vi "GVSGet Window Title Message.vi"(10 "No":i32, 11 "Kind":string) -> (0 "Control Label Off":string[](array[string]), 1 "Control Label On":string[](array[string]), 2 "Unicode String":string, 3 "Multibyte String":string, 4 "Control Name":string[](array[string]), 6 "Tip Strip":string[](array[string]))   [LabVIEW 2013]
panel:
  # "Get Window Title Message."
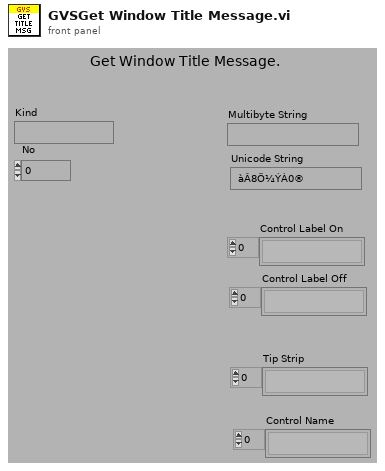
[diagram p1: front panel]
types:
  T1 = enum32{"English", "Chinese", "Korean", "Japanese", "Russian", "Chinese traditional"}
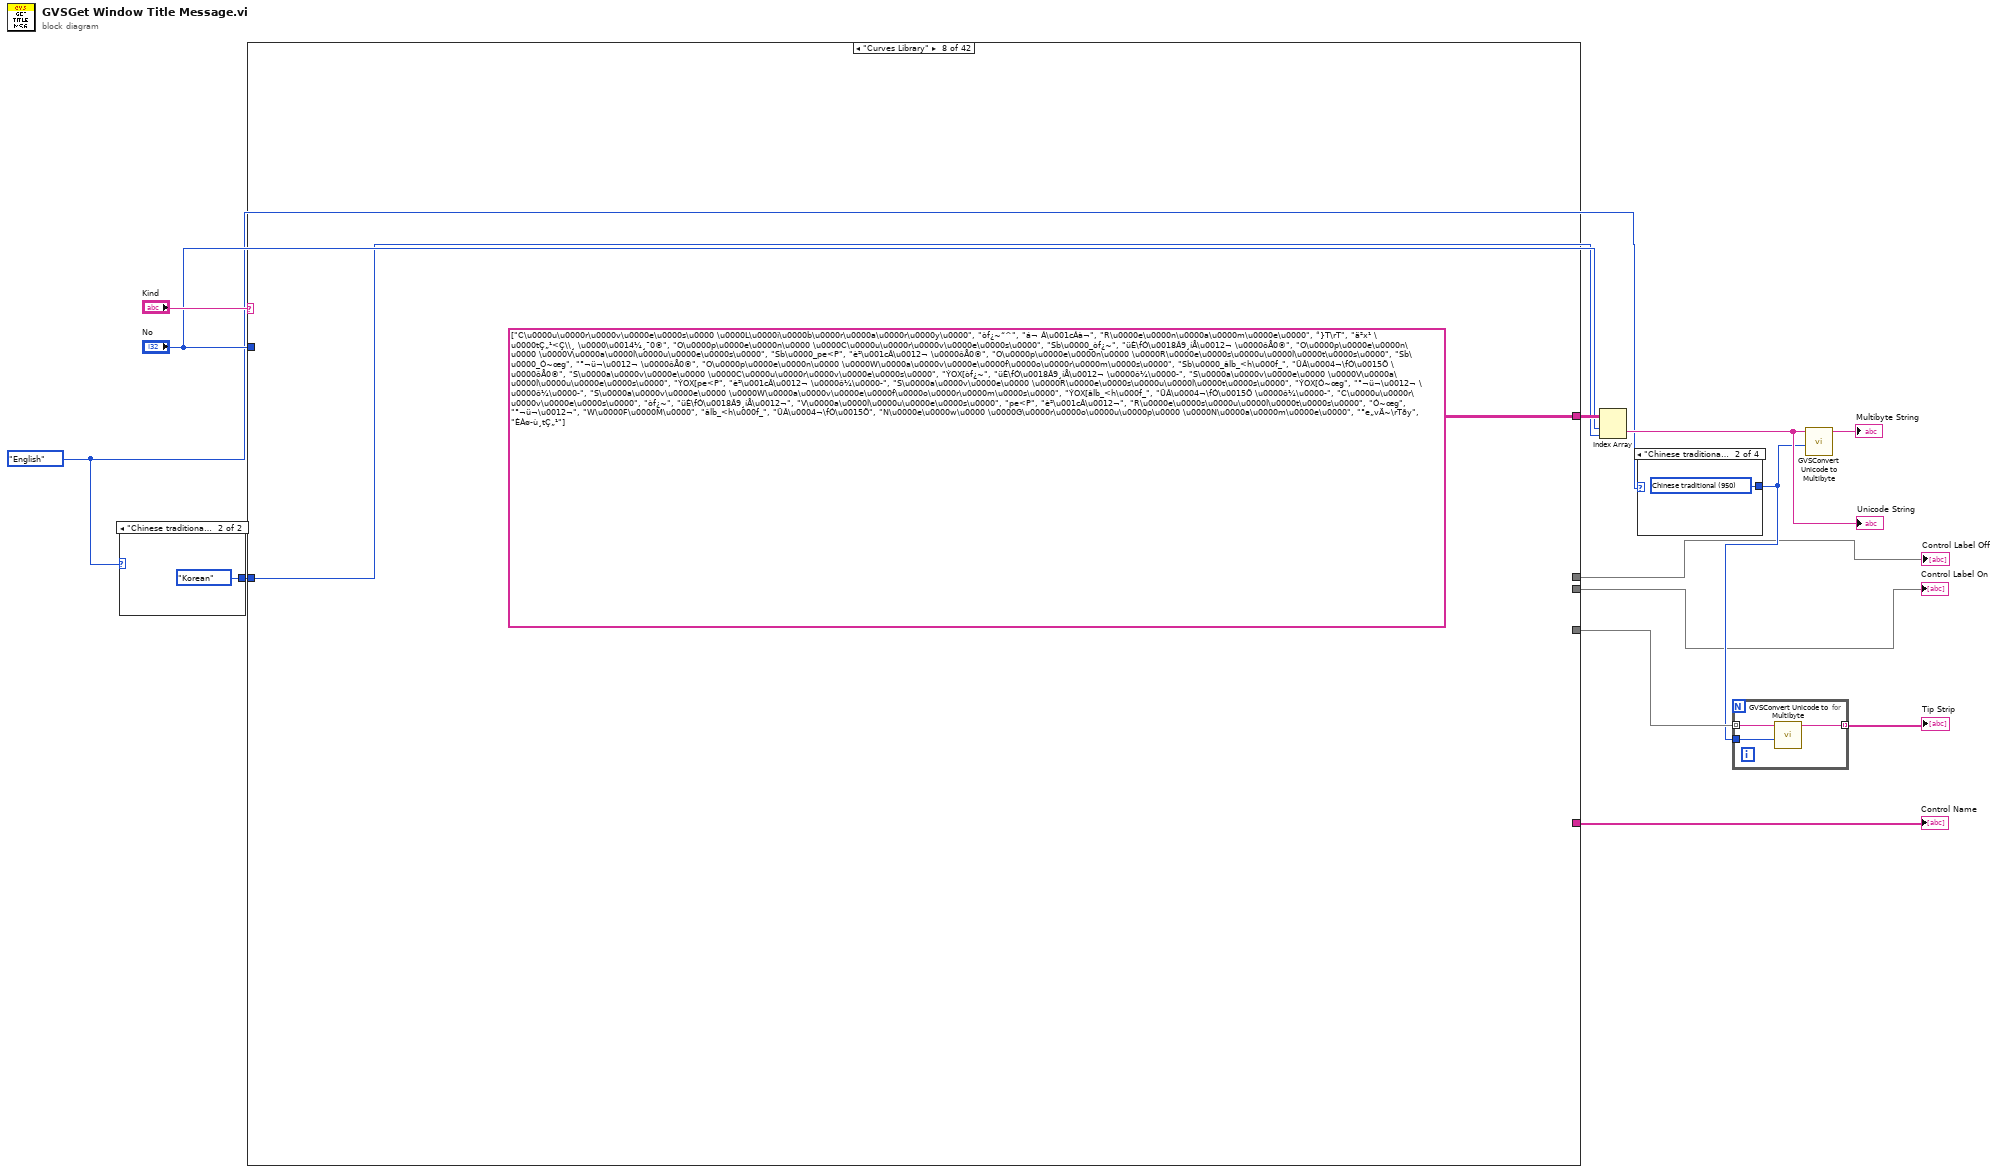
[diagram p0: block diagram]
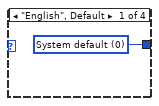
[diagram p3: hidden frame]
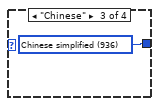
[diagram p4: hidden frame]
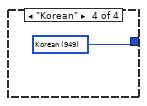
[diagram p5: hidden frame]
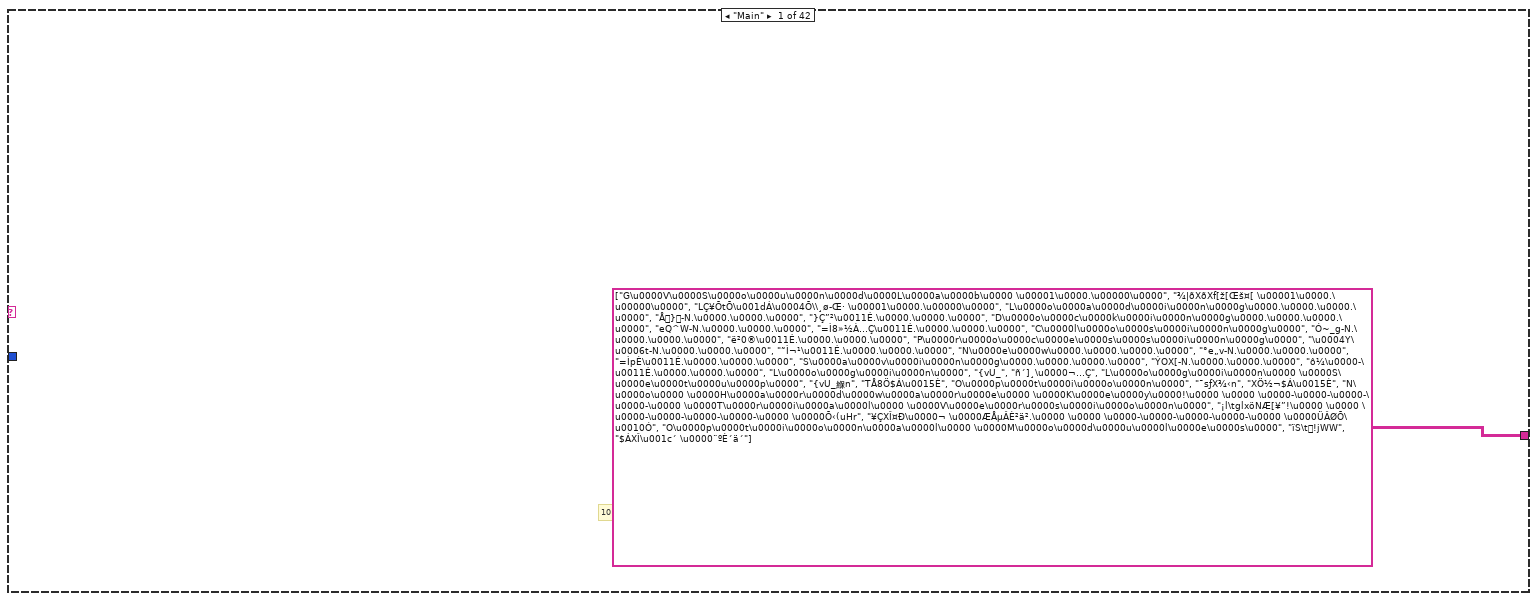
[diagram p6: hidden frame]
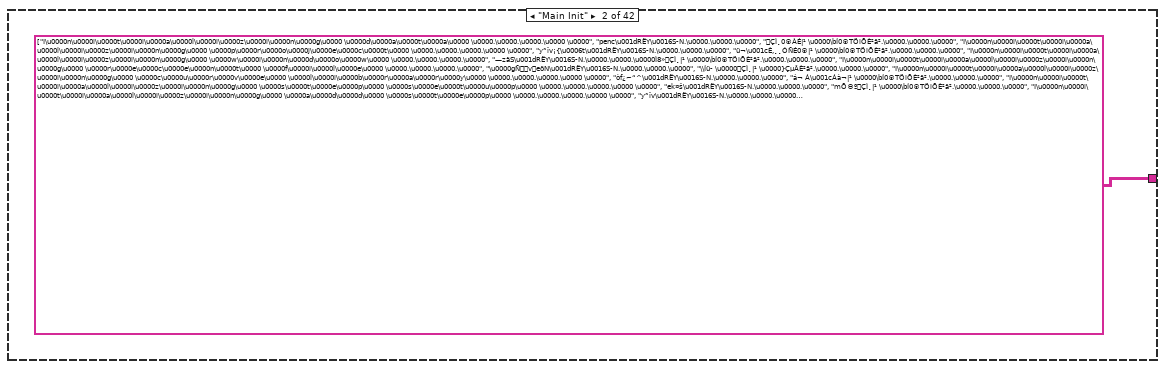
[diagram p7: hidden frame]
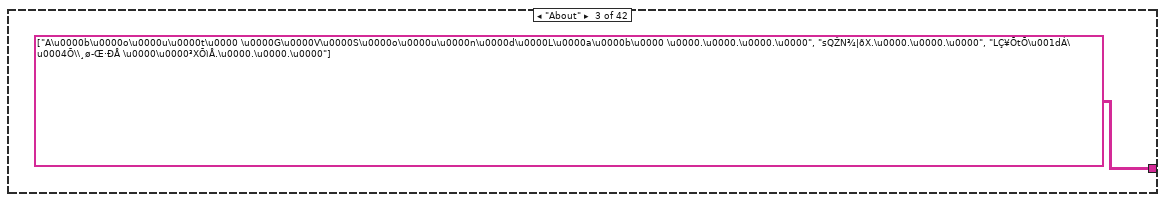
[diagram p8: hidden frame]
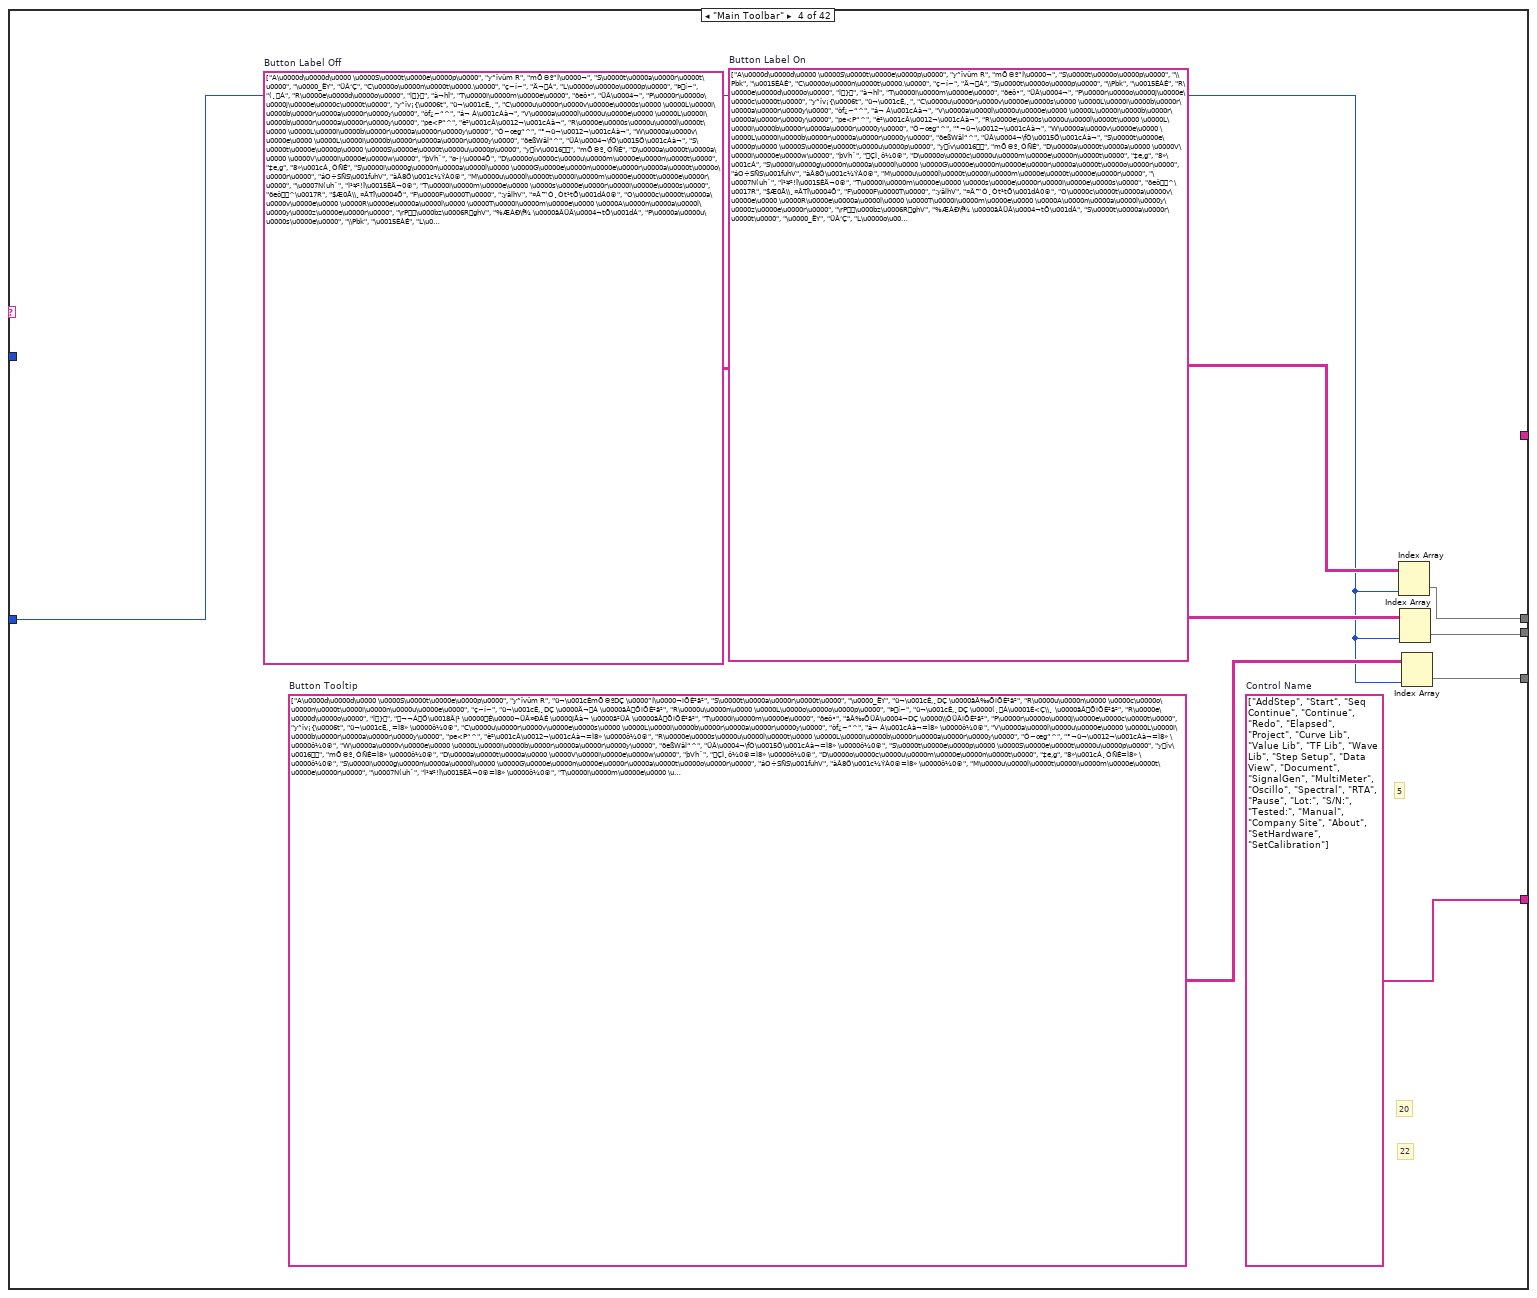
[diagram p9: hidden frame]
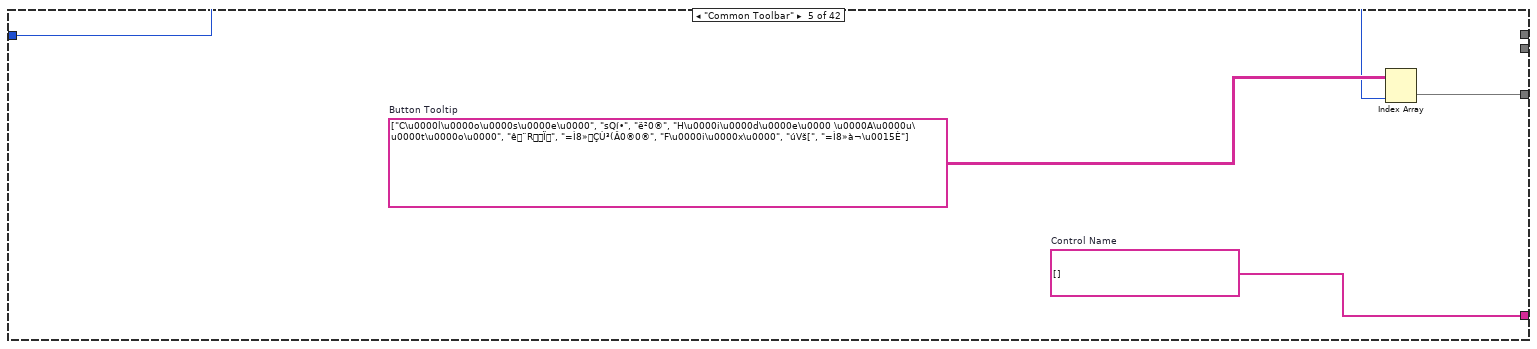
[diagram p10: hidden frame]
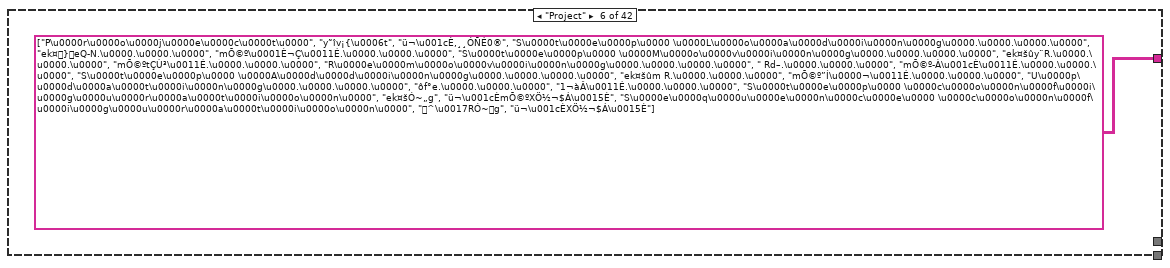
[diagram p11: hidden frame]
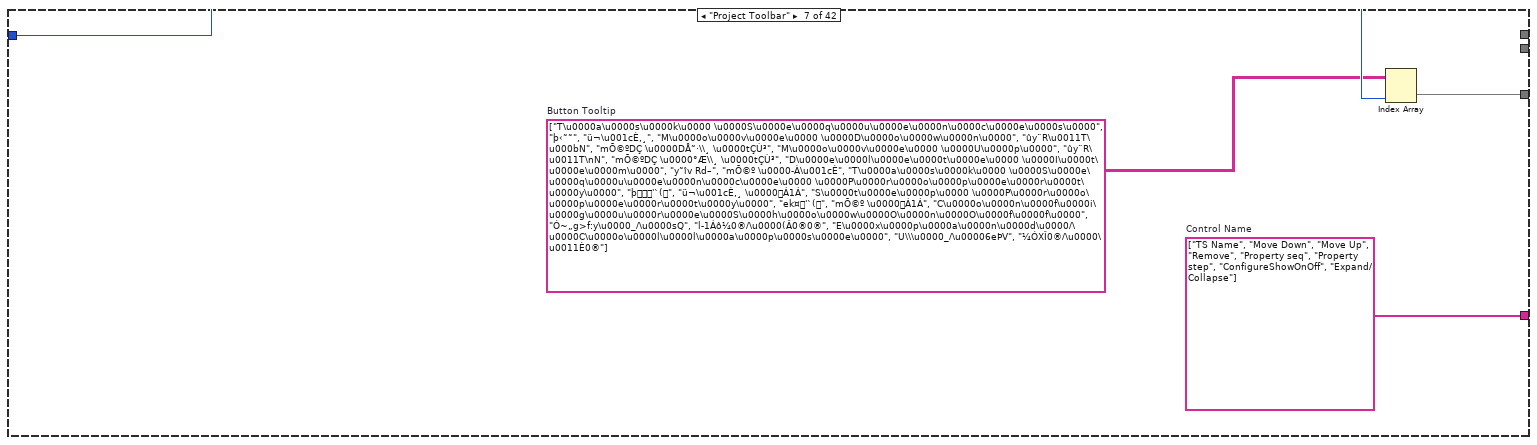
[diagram p12: hidden frame]
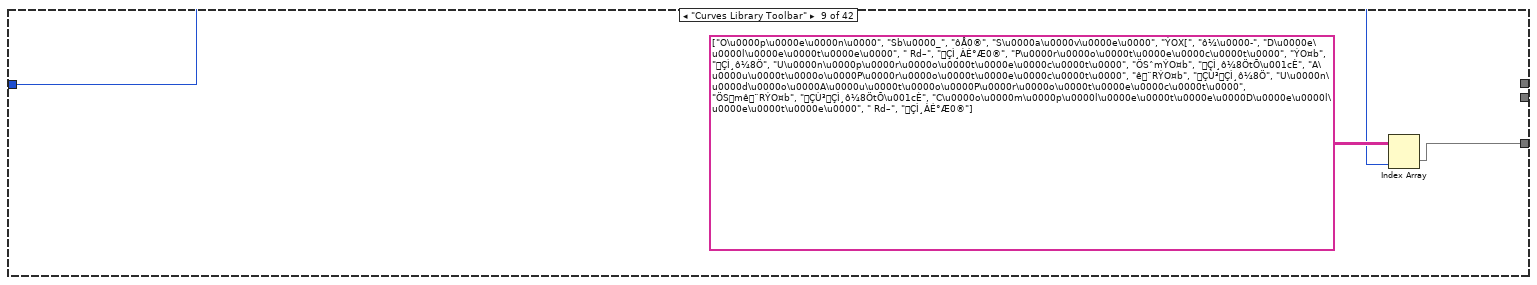
[diagram p13: hidden frame]
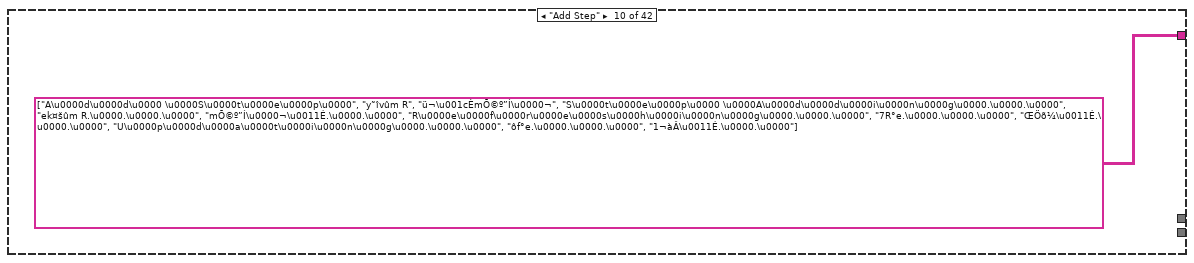
[diagram p14: hidden frame]
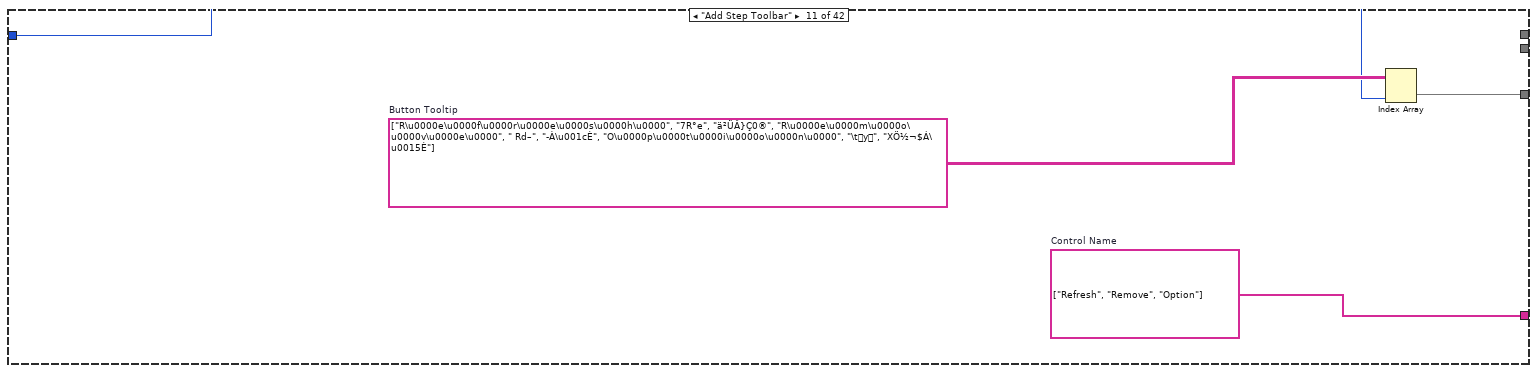
[diagram p15: hidden frame]
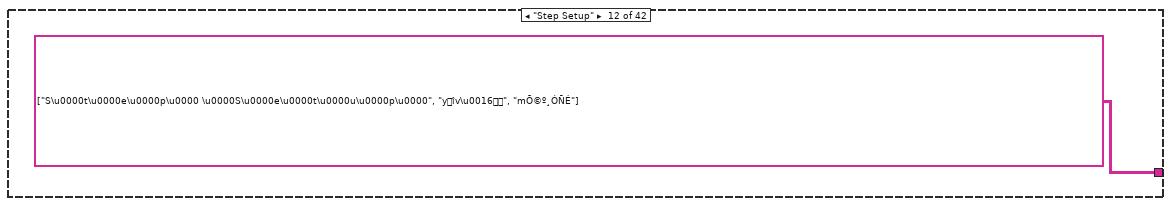
[diagram p16: hidden frame]
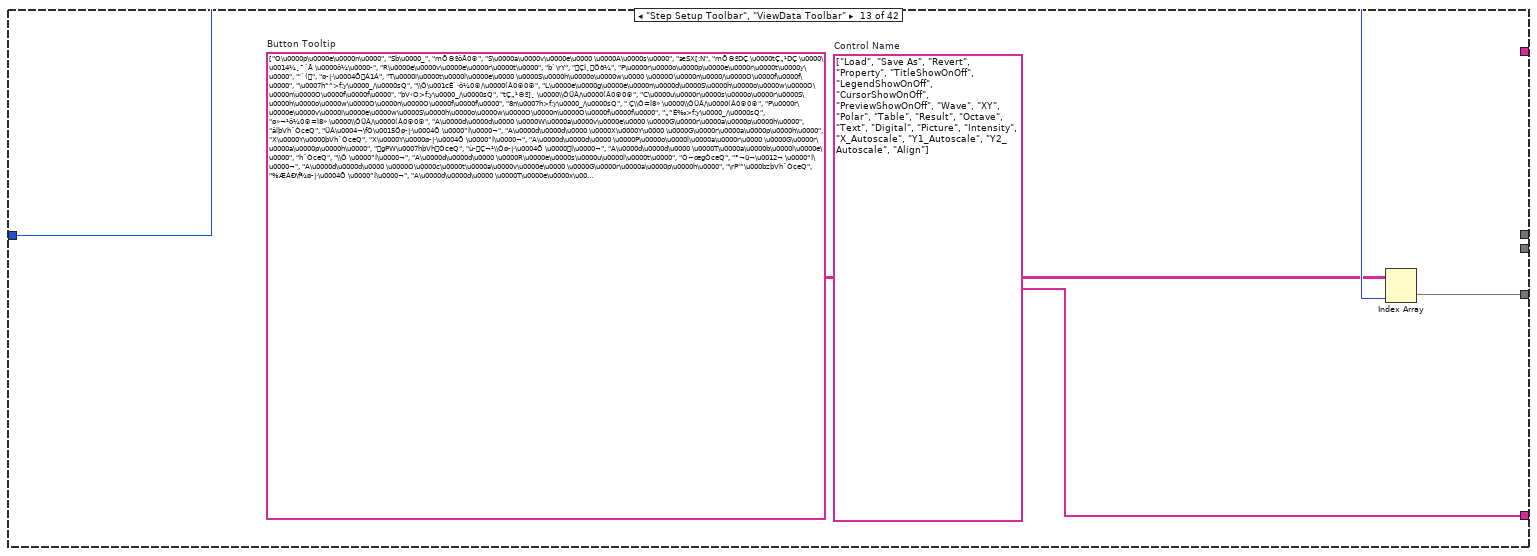
[diagram p17: hidden frame]
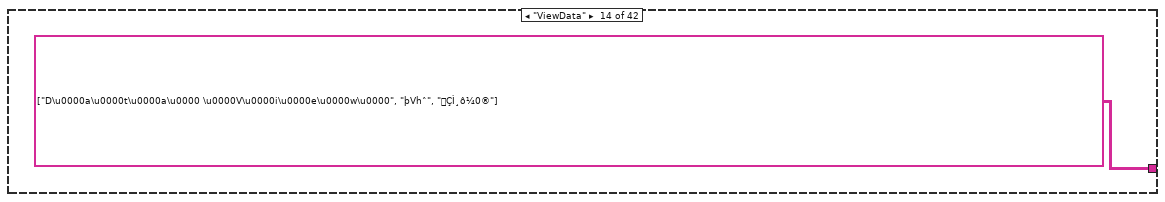
[diagram p18: hidden frame]
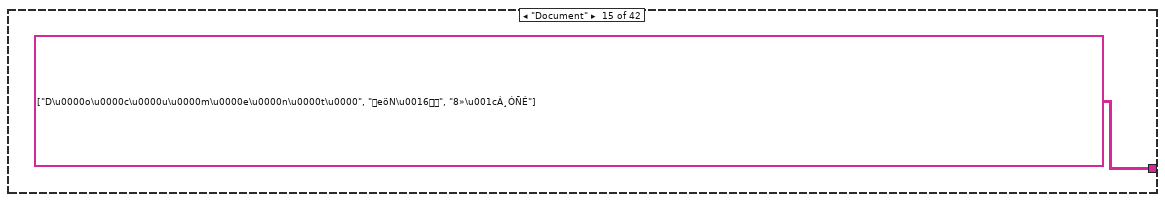
[diagram p19: hidden frame]
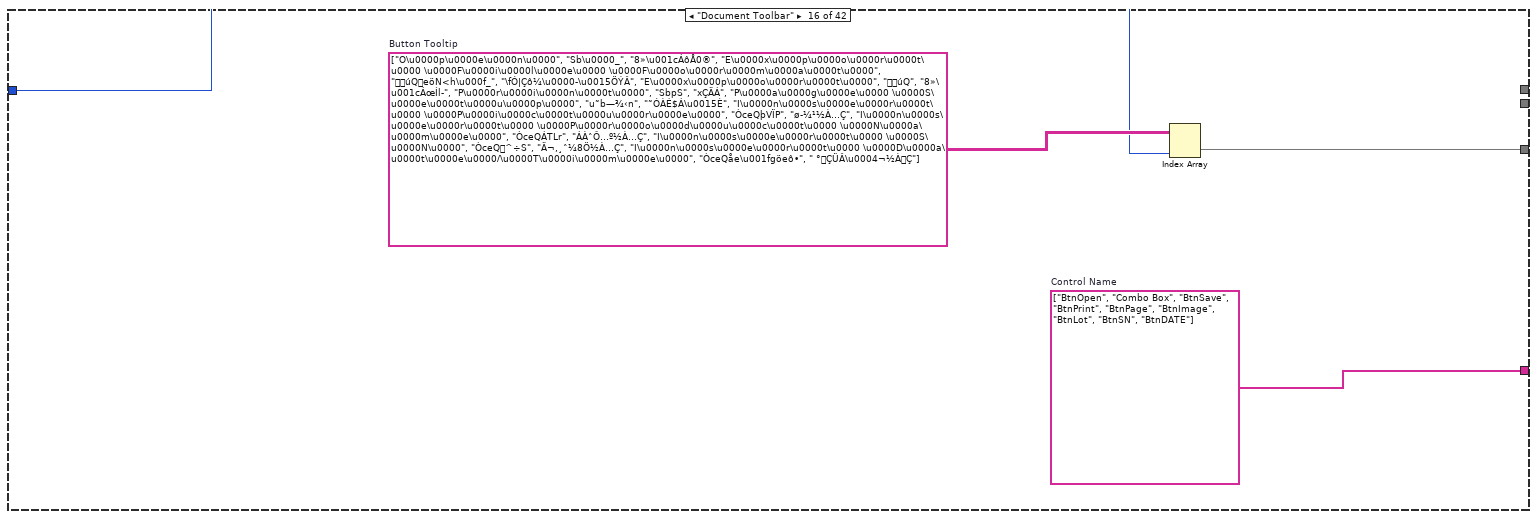
[diagram p20: hidden frame]
diagram:
  w1 = T1."English" ("Language")
  n1 = case shown="\"Chinese traditional\"" w1 {
    selector: w1 -> [w14 _]
    tunnel: [w14 T1."Korean" ("Language")] -> w2
    frame "English", Default {
    }
    frame "Chinese traditional" {
    }
  }
  n2 = case shown="\"Curves Library\"" "Kind" {
    tunnel: [string[][] [["G\u0000V\u0000S\u0000o\u0000u\u0000n\u0000d\u0000L\u0000a\u0000b\u0000 \u00001\u0000.\u00000\u0000", "¾|ðXðXf[ž[Œš¤[ \u00001\u0000.\u00000\u0000", "LÇ¥ÕtÕ\u001dÁ\u0004Õ\\¸ø­Œ· \u00001\u0000.\u00000\u0000"], ["L\u0000o\u0000a\u0000d\u0000i\u0000n\u0000g\u0000.\u0000.\u0000.\u0000", "Å}-N.\u0000.\u0000.\u0000", "}Ç”²\u0011É.\u0000.\u0000.\u0000"], ["D\u0000o\u0000c\u0000k\u0000i\u0000n\u0000g\u0000.\u0000.\u0000.\u0000", "eQ^W-N.\u0000.\u0000.\u0000", "=Ì8»½À…Ç\u0011É.\u0000.\u0000.\u0000"], ["C\u0000l\u0000o\u0000s\u0000i\u0000n\u0000g\u0000", "Ó~_g-N.\u0000.\u0000.\u0000", "ë²0®\u0011É.\u0000.\u0000.\u0000"], ["P\u0000r\u0000o\u0000c\u0000e\u0000s\u0000s\u0000i\u0000n\u0000g\u0000", "\u0004Y\u0006t-N.\u0000.\u0000.\u0000", "˜Ì¬¹\u0011É.\u0000.\u0000.\u0000"], ["N\u0000e\u0000w\u0000.\u0000.\u0000.\u0000", "°e„v-N.\u0000.\u0000.\u0000", "=ÌpÈ\u0011É.\u0000.\u0000.\u0000"], ["S\u0000a\u0000v\u0000i\u0000n\u0000g\u0000.\u0000.\u0000.\u0000", "ÝOX[-N.\u0000.\u0000.\u0000", "ô¼\u0000­\u0011É.\u0000.\u0000.\u0000"], ["L\u0000o\u0000g\u0000i\u0000n\u0000", "{vU_", "ñ´]¸\u0000¬…Ç"], ["L\u0000o\u0000g\u0000i\u0000n\u0000 \u0000S\u0000e\u0000t\u0000u\u0000p\u0000", "{vU_緥n", "TÅ8Ö$Á\u0015È"], ["O\u0000p\u0000t\u0000i\u0000o\u0000n\u0000", "¯sƒX¾‹n", "XÖ½¬$Á\u0015È"], ["N\u0000o\u0000 \u0000H\u0000a\u0000r\u0000d\u0000w\u0000a\u0000r\u0000e\u0000 \u0000K\u0000e\u0000y\u0000!\u0000 \u0000 \u0000-\u0000-\u0000-\u0000-\u0000 \u0000T\u0000r\u0000i\u0000a\u0000l\u0000 \u0000V\u0000e\u0000r\u0000s\u0000i\u0000o\u0000n\u0000", "¡l\tglxöNÆ[¥”!\u0000 \u0000 \u0000-\u0000-\u0000-\u0000-\u0000 \u0000Õ‹(uHr", "¥ÇXÎ¤Ð\u0000¬ \u0000ÆÅµÂÈ²ä².\u0000 \u0000 \u0000-\u0000-\u0000-\u0000-\u0000 \u0000ÜÂØÕ\u0010Ó"], ["O\u0000p\u0000t\u0000i\u0000o\u0000n\u0000a\u0000l\u0000 \u0000M\u0000o\u0000d\u0000u\u0000l\u0000e\u0000s\u0000", "ïS\t!jWW", "$ÁXÎ\u001c´ \u0000¨ºÈ´ä´"]] string[][] [["I\u0000n\u0000i\u0000t\u0000i\u0000a\u0000l\u0000i\u0000z\u0000i\u0000n\u0000g\u0000 \u0000d\u0000a\u0000t\u0000a\u0000 \u0000.\u0000.\u0000.\u0000 \u0000", "penc\u001dRËY\u0016S-N.\u0000.\u0000.\u0000", "ÇÌ¸0®ÀÉ|¹ \u0000\bÍ0®TÖiÕÈ²ä².\u0000.\u0000.\u0000"], ["I\u0000n\u0000i\u0000t\u0000i\u0000a\u0000l\u0000i\u0000z\u0000i\u0000n\u0000g\u0000 \u0000p\u0000r\u0000o\u0000j\u0000e\u0000c\u0000t\u0000 \u0000.\u0000.\u0000.\u0000 \u0000", "y˜îv¡{\u0006t\u001dRËY\u0016S-N.\u0000.\u0000.\u0000", "ü¬\u001cÈ,¸¸ÓÑÉ0®|¹ \u0000\bÍ0®TÖiÕÈ²ä².\u0000.\u0000.\u0000"], ["I\u0000n\u0000i\u0000t\u0000i\u0000a\u0000l\u0000i\u0000z\u0000i\u0000n\u0000g\u0000 \u0000w\u0000i\u0000n\u0000d\u0000o\u0000w\u0000 \u0000.\u0000.\u0000.\u0000", "—zãS\u001dRËY\u0016S-N.\u0000.\u0000.\u0000", "=Ì8»ÇÌ¸|¹ \u0000\bÍ0®TÖiÕÈ²ä².\u0000.\u0000.\u0000"], ["I\u0000n\u0000i\u0000t\u0000i\u0000a\u0000l\u0000i\u0000z\u0000i\u0000n\u0000g\u0000 \u0000r\u0000e\u0000c\u0000e\u0000n\u0000t\u0000 \u0000f\u0000i\u0000l\u0000e\u0000 \u0000.\u0000.\u0000.\u0000", "\u0000gÑveöN\u001dRËY\u0016S-N.\u0000.\u0000.\u0000", "\\Íü­ \u0000ÇÌ¸|¹ \u0000}ÇµÂÈ²ä².\u0000.\u0000.\u0000"], ["I\u0000n\u0000i\u0000t\u0000i\u0000a\u0000l\u0000i\u0000z\u0000i\u0000n\u0000g\u0000 \u0000c\u0000u\u0000r\u0000v\u0000e\u0000 \u0000l\u0000i\u0000b\u0000r\u0000a\u0000r\u0000y\u0000 \u0000.\u0000.\u0000.\u0000 \u0000", "òf¿~“^\u001dRËY\u0016S-N.\u0000.\u0000.\u0000", "á¬ Á\u001cÁà¬|¹ \u0000\bÍ0®TÖiÕÈ²ä².\u0000.\u0000.\u0000"], ["I\u0000n\u0000i\u0000t\u0000i\u0000a\u0000l\u0000i\u0000z\u0000i\u0000n\u0000g\u0000 \u0000s\u0000t\u0000e\u0000p\u0000 \u0000s\u0000e\u0000t\u0000u\u0000p\u0000 \u0000.\u0000.\u0000.\u0000 \u0000", "ek¤š\u001dRËY\u0016S-N.\u0000.\u0000.\u0000", "mÕ©ºÇÌ¸|¹ \u0000\bÍ0®TÖiÕÈ²ä².\u0000.\u0000.\u0000"], ["I\u0000n\u0000i\u0000t\u0000i\u0000a\u0000l\u0000i\u0000z\u0000i\u0000n\u0000g\u0000 \u0000a\u0000d\u0000d\u0000 \u0000s\u0000t\u0000e\u0000p\u0000 \u0000.\u0000.\u0000.\u0000 \u0000", "y˜îv\u001dRËY\u0016S-N.\u0000.\u0000.\u0000", "mÕ©ºÍ\u0000¬ÇÌ¸|¹ \u0000\u0001È¬ÇiÕÈ²ä².\u0000.\u0000.\u0000"], ["I\u0000n\u0000i\u0000t\u0000i\u0000a\u0000l\u0000i\u0000z\u0000i\u0000n\u0000g\u0000 \u0000t\u0000a\u0000s\u0000k\u0000 \u0000s\u0000e\u0000q\u0000u\u0000e\u0000n\u0000c\u0000e\u0000 \u0000.\u0000.\u0000.\u0000", "^\u0017R\u001dRËY\u0016S-N.\u0000.\u0000.\u0000", "ü¬\u001cÈ,¸DÇ \u0000\bÍ0®TÖiÕÈ²ä².\u0000.\u0000.\u0000"], ["I\u0000n\u0000i\u0000t\u0000i\u0000a\u0000l\u0000i\u0000z\u0000i\u0000n\u0000g\u0000 \u0000v\u0000i\u0000r\u0000t\u0000u\u0000a\u0000l\u0000 \u0000d\u0000a\u0000t\u0000a\u0000 \u0000.\u0000.\u0000.\u0000", "—zãS\u001dRËY\u0016S-N.\u0000.\u0000.\u0000", "\u0000¬ÁÀ=Ì8»ÇÌ¸|¹ \u0000\u0001È¬ÇiÕÈ²ä².\u0000.\u0000.\u0000"], ["I\u0000n\u0000i\u0000t\u0000i\u0000a\u0000l\u0000i\u0000z\u0000i\u0000n\u0000g\u0000 \u0000O\u0000p\u0000e\u0000r\u0000a\u0000t\u0000o\u0000r\u0000 \u0000.\u0000.\u0000.\u0000 \u0000", "Íd\\O\u001dRËY\u0016S-N.\u0000.\u0000.\u0000", "äÂÜÂ\u0004¬Ä³l­|¹ \u0000\bÍ0®TÖiÕÈ²ä².\u0000.\u0000.\u0000"], ["L\u0000o\u0000a\u0000d\u0000i\u0000n\u0000g\u0000 \u0000m\u0000a\u0000i\u0000n\u0000 \u0000w\u0000i\u0000n\u0000d\u0000o\u0000w\u0000 \u0000.\u0000.\u0000.\u0000", ";N—zãS\u001dRËY\u0016S-N.\u0000.\u0000.\u0000", "üÈ\u0004Õ\\¸ø­Œ·DÇ \u0000\u0001È¬ÇXÕà¬ˆÇµÂÈ²ä².\u0000.\u0000.\u0000"], ["L\u0000o\u0000a\u0000d\u0000i\u0000n\u0000g\u0000 \u0000m\u0000a\u0000i\u0000n\u0000 \u0000w\u0000i\u0000n\u0000d\u0000o\u0000w\u0000 \u0000.\u0000 \u0000.\u0000", ";N—zãS\u001dRËY\u0016S-N.\u0000 \u0000.\u0000", "üÈ\u0004Õ\\¸ø­Œ·DÇ \u0000\u0001È¬ÇXÕà¬ˆÇµÂÈ²ä².\u0000 \u0000.\u0000"], ["L\u0000o\u0000a\u0000d\u0000i\u0000n\u0000g\u0000 \u0000m\u0000a\u0000i\u0000n\u0000 \u0000w\u0000i\u0000n\u0000d\u0000o\u0000w\u0000 \u0000.\u0000.\u0000 \u0000", ";N—zãS\u001dRËY\u0016S-N.\u0000.\u0000 \u0000", "üÈ\u0004Õ\\¸ø­Œ·DÇ \u0000\u0001È¬ÇXÕà¬ˆÇµÂÈ²ä².\u0000.\u0000 \u0000"]] string[][] [["A\u0000b\u0000o\u0000u\u0000t\u0000 \u0000G\u0000V\u0000S\u0000o\u0000u\u0000n\u0000d\u0000L\u0000a\u0000b\u0000 \u0000.\u0000.\u0000.\u0000", "sQŽN¾|ðX.\u0000.\u0000.\u0000", "LÇ¥ÕtÕ\u001dÁ\u0004Õ\\¸ø­Œ·ÐÅ \u0000\u0000³XÕìÅ.\u0000.\u0000.\u0000"]] _ _ string[][] [["P\u0000r\u0000o\u0000j\u0000e\u0000c\u0000t\u0000", "y˜îv¡{\u0006t", "ü¬\u001cÈ,¸¸ÓÑÉ0®"], ["S\u0000t\u0000e\u0000p\u0000 \u0000L\u0000o\u0000a\u0000d\u0000i\u0000n\u0000g\u0000.\u0000.\u0000.\u0000", "ek¤}eQ-N.\u0000.\u0000.\u0000", "mÕ©º\u0001È¬Ç\u0011É.\u0000.\u0000.\u0000"], ["S\u0000t\u0000e\u0000p\u0000 \u0000M\u0000o\u0000v\u0000i\u0000n\u0000g\u0000.\u0000.\u0000.\u0000", "ek¤šûy¨R.\u0000.\u0000.\u0000", "mÕ©ºtÇÙ³\u0011É.\u0000.\u0000.\u0000"], ["R\u0000e\u0000m\u0000o\u0000v\u0000i\u0000n\u0000g\u0000.\u0000.\u0000.\u0000", " Rd–.\u0000.\u0000.\u0000", "mÕ©º­À\u001cÈ\u0011É.\u0000.\u0000.\u0000"], ["S\u0000t\u0000e\u0000p\u0000 \u0000A\u0000d\u0000d\u0000i\u0000n\u0000g\u0000.\u0000.\u0000.\u0000", "ek¤šûm R.\u0000.\u0000.\u0000", "mÕ©º”Í\u0000¬\u0011É.\u0000.\u0000.\u0000"], ["U\u0000p\u0000d\u0000a\u0000t\u0000i\u0000n\u0000g\u0000.\u0000.\u0000.\u0000", "ôf°e.\u0000.\u0000.\u0000", "1¬àÂ\u0011É.\u0000.\u0000.\u0000"], ["S\u0000t\u0000e\u0000p\u0000 \u0000c\u0000o\u0000n\u0000f\u0000i\u0000g\u0000u\u0000r\u0000a\u0000t\u0000i\u0000o\u0000n\u0000", "ek¤šÓ~„g", "ü¬\u001cÈmÕ©ºXÖ½¬$Á\u0015È"], ["S\u0000e\u0000q\u0000u\u0000e\u0000n\u0000c\u0000e\u0000 \u0000c\u0000o\u0000n\u0000f\u0000i\u0000g\u0000u\u0000r\u0000a\u0000t\u0000i\u0000o\u0000n\u0000", "^\u0017RÓ~g", "ü¬\u001cÈXÖ½¬$Á\u0015È"]] _ string[][] [["C\u0000u\u0000r\u0000v\u0000e\u0000s\u0000 \u0000L\u0000i\u0000b\u0000r\u0000a\u0000r\u0000y\u0000", "òf¿~“^", "á¬ Á\u001cÁà¬"], ["R\u0000e\u0000n\u0000a\u0000m\u0000e\u0000", "͑}T\rT", "ä²x¹ \u0000tÇ„¹<Ç\\¸ \u0000\u0014¼¸¯0®"], ["O\u0000p\u0000e\u0000n\u0000 \u0000C\u0000u\u0000r\u0000v\u0000e\u0000s\u0000", "Sb\u0000_òf¿~", "üÈ\fÓ\u0018Â9¸íÅ\u0012¬ \u0000ôÅ0®"], ["O\u0000p\u0000e\u0000n\u0000 \u0000V\u0000a\u0000l\u0000u\u0000e\u0000s\u0000", "Sb\u0000_pe<P", "è²\u001cÂ\u0012¬ \u0000ôÅ0®"], ["O\u0000p\u0000e\u0000n\u0000 \u0000R\u0000e\u0000s\u0000u\u0000l\u0000t\u0000s\u0000", "Sb\u0000_Ó~œg", "°¬ü¬\u0012¬ \u0000ôÅ0®"], ["O\u0000p\u0000e\u0000n\u0000 \u0000W\u0000a\u0000v\u0000e\u0000f\u0000o\u0000r\u0000m\u0000s\u0000", "Sb\u0000_âlb_<h\u000f_", "ÜÂ\u0004¬\fÓ\u0015Ö \u0000ôÅ0®"], ["S\u0000a\u0000v\u0000e\u0000 \u0000C\u0000u\u0000r\u0000v\u0000e\u0000s\u0000", "ÝOX[òf¿~", "üÈ\fÓ\u0018Â9¸íÅ\u0012¬ \u0000ô¼\u0000­"], ["S\u0000a\u0000v\u0000e\u0000 \u0000V\u0000a\u0000l\u0000u\u0000e\u0000s\u0000", "ÝOX[pe<P", "è²\u001cÂ\u0012¬ \u0000ô¼\u0000­"], ["S\u0000a\u0000v\u0000e\u0000 \u0000R\u0000e\u0000s\u0000u\u0000l\u0000t\u0000s\u0000", "ÝOX[Ó~œg", "°¬ü¬\u0012¬ \u0000ô¼\u0000­"], ["S\u0000a\u0000v\u0000e\u0000 \u0000W\u0000a\u0000v\u0000e\u0000f\u0000o\u0000r\u0000m\u0000s\u0000", "ÝOX[âlb_<h\u000f_", "ÜÂ\u0004¬\fÓ\u0015Ö \u0000ô¼\u0000­"], ["C\u0000u\u0000r\u0000v\u0000e\u0000s\u0000", "òf¿~", "üÈ\fÓ\u0018Â9¸íÅ\u0012¬"], ["V\u0000a\u0000l\u0000u\u0000e\u0000s\u0000", "pe<P", "è²\u001cÂ\u0012¬"], ["R\u0000e\u0000s\u0000u\u0000l\u0000t\u0000s\u0000", "Ó~œg", "°¬ü¬\u0012¬"], ["W\u0000F\u0000M\u0000", "âlb_<h\u000f_", "ÜÂ\u0004¬\fÓ\u0015Ö"], ["N\u0000e\u0000w\u0000 \u0000G\u0000r\u0000o\u0000u\u0000p\u0000 \u0000N\u0000a\u0000m\u0000e\u0000", "°e„vÄ~\rTðy", "ÈÀø­ù¸tÇ„¹"]] _ string[][] [["A\u0000d\u0000d\u0000 \u0000S\u0000t\u0000e\u0000p\u0000", "y˜îvûm R", "ü¬\u001cÈmÕ©º”Í\u0000¬"], ["S\u0000t\u0000e\u0000p\u0000 \u0000A\u0000d\u0000d\u0000i\u0000n\u0000g\u0000.\u0000.\u0000", "ek¤šûm R.\u0000.\u0000.\u0000", "mÕ©º”Í\u0000¬\u0011É.\u0000.\u0000"], ["R\u0000e\u0000f\u0000r\u0000e\u0000s\u0000h\u0000i\u0000n\u0000g\u0000.\u0000.\u0000", "7R°e.\u0000.\u0000.\u0000", "ŒÖõ¼\u0011É.\u0000.\u0000"], ["U\u0000p\u0000d\u0000a\u0000t\u0000i\u0000n\u0000g\u0000.\u0000.\u0000", "ôf°e.\u0000.\u0000.\u0000", "1¬àÂ\u0011É.\u0000.\u0000"]] _ string[][] [["S\u0000t\u0000e\u0000p\u0000 \u0000S\u0000e\u0000t\u0000u\u0000p\u0000", "yîv\u0016", "mÕ©º¸ÓÑÉ"]] _ string[][] [["D\u0000a\u0000t\u0000a\u0000 \u0000V\u0000i\u0000e\u0000w\u0000", "þVhˆ", "ÇÌ¸ô¼0®"]] string[][] [["D\u0000o\u0000c\u0000u\u0000m\u0000e\u0000n\u0000t\u0000", "eöN\u0016", "8»\u001cÁ¸ÓÑÉ"]] _ string[][] [["R\u0000u\u0000n\u0000 \u0000P\u0000r\u0000o\u0000j\u0000e\u0000c\u0000t\u0000", "yîvÐL", "ü¬\u001cÈ,¸ \u0000äÂ‰Õ"]] string[][] [["W\u0000a\u0000v\u0000e\u0000 \u0000G\u0000r\u0000a\u0000p\u0000h\u0000", "âlþVhˆ", "ÜÂ\u0004¬\fÓ\u0015Öø­|·\u0004Õ"], ["W\u0000a\u0000v\u0000e\u0000 \u0000G\u0000r\u0000a\u0000p\u0000h\u0000 \u0000P\u0000r\u0000o\u0000p\u0000e\u0000r\u0000t\u0000y\u0000", "âlþVhˆ^\\'`", "ÜÂ\u0004¬\fÓ\u0015Öø­|·\u0004ÕÁ1Á"]] string[][] [["X\u0000Y\u0000 \u0000G\u0000r\u0000a\u0000p\u0000h\u0000", "X\u0000Y\u0000þVhˆ", "X\u0000Y\u0000ø­|·\u0004Õ"], ["X\u0000Y\u0000 \u0000G\u0000r\u0000a\u0000p\u0000h\u0000 \u0000P\u0000r\u0000o\u0000p\u0000e\u0000r\u0000t\u0000y\u0000", "X\u0000Y\u0000þVhˆ^\\'`", "X\u0000Y\u0000ø­|·\u0004ÕÁ1Á"]] string[][] [["D\u0000i\u0000g\u0000i\u0000t\u0000a\u0000l\u0000 \u0000G\u0000r\u0000a\u0000p\u0000h\u0000", "peW[þVhˆ", "\u0018ÂÇàÂ8Öø­|·\u0004Õ"], ["D\u0000i\u0000g\u0000i\u0000t\u0000a\u0000l\u0000 \u0000G\u0000r\u0000a\u0000p\u0000h\u0000 \u0000P\u0000r\u0000o\u0000p\u0000e\u0000r\u0000t\u0000y\u0000", "peW[þVhˆ^\\'`", "\u0018ÂÇàÂ8Öø­|·\u0004ÕÁ1Á"]] string[][] [["O\u0000c\u0000t\u0000a\u0000v\u0000e\u0000 \u0000G\u0000r\u0000a\u0000p\u0000h\u0000", "\rP‘˜\u000bzþVhˆ", "%ÆÀÐ\f¾ø­|·\u0004Õ"], ["O\u0000c\u0000t\u0000a\u0000v\u0000e\u0000 \u0000G\u0000r\u0000a\u0000p\u0000h\u0000 \u0000P\u0000r\u0000o\u0000p\u0000e\u0000r\u0000t\u0000y\u0000", "\rP‘˜\u000bzþVhˆ^\\'`", "%ÆÀÐ\f¾ø­|·\u0004ÕÁ1Á"]] string[][] [["P\u0000o\u0000l\u0000a\u0000r\u0000 \u0000G\u0000r\u0000a\u0000p\u0000h\u0000", "gPW\u0007hþVh", "ù­Ç¬¹\\Ôø­|·\u0004Õ"], ["P\u0000o\u0000l\u0000a\u0000r\u0000 \u0000G\u0000r\u0000a\u0000p\u0000h\u0000 \u0000P\u0000r\u0000o\u0000p\u0000e\u0000r\u0000t\u0000y\u0000 \u0000", "gPW\u0007hþVh^\\'`", "ù­Ç¬¹\\Ôø­|·\u0004ÕÁ1Á"]] string[][] [["T\u0000e\u0000x\u0000t\u0000", ",g‡e", "ø¼8»"], ["T\u0000e\u0000x\u0000t\u0000 \u0000P\u0000r\u0000o\u0000p\u0000e\u0000r\u0000t\u0000y\u0000", ",g‡e^\\'`", "ø¼8»Á1Á"]] string[][] [["T\u0000a\u0000b\u0000l\u0000e\u0000 \u0000G\u0000r\u0000a\u0000p\u0000h\u0000", "hˆ", "\\Ô"], ["T\u0000a\u0000b\u0000l\u0000e\u0000 \u0000G\u0000r\u0000a\u0000p\u0000h\u0000 \u0000P\u0000r\u0000o\u0000p\u0000e\u0000r\u0000t\u0000y\u0000", "hˆ^\\'`", "\\ÔÁ1Á"]] string[][] [["P\u0000i\u0000c\u0000t\u0000u\u0000r\u0000e\u0000 \u0000G\u0000r\u0000a\u0000p\u0000h\u0000", "þVÏP", "ø­¼¹"], ["P\u0000i\u0000c\u0000t\u0000u\u0000r\u0000e\u0000 \u0000G\u0000r\u0000a\u0000p\u0000h\u0000 \u0000P\u0000r\u0000o\u0000p\u0000e\u0000r\u0000t\u0000y\u0000", "þVÏP^\\'`", "ø­¼¹Á1Á"]] string[][] [["R\u0000e\u0000s\u0000u\u0000l\u0000t\u0000 \u0000G\u0000r\u0000a\u0000p\u0000h\u0000", "Ó~œg", "°¬ü¬\u0012¬"], ["R\u0000e\u0000s\u0000u\u0000l\u0000t\u0000 \u0000G\u0000r\u0000a\u0000p\u0000h\u0000 \u0000P\u0000r\u0000o\u0000p\u0000e\u0000r\u0000t\u0000y\u0000", "Ó~œg^\\'`", "°¬ü¬\u0012¬Á1Á"]] string[][] [["I\u0000n\u0000t\u0000e\u0000n\u0000s\u0000i\u0000t\u0000y\u0000 \u0000G\u0000r\u0000a\u0000p\u0000h\u0000", "Æ[¦^þVhˆ", "\u0000¼Ä³ø­|·\u0004Õ"], ["I\u0000n\u0000t\u0000e\u0000n\u0000s\u0000i\u0000t\u0000y\u0000 \u0000G\u0000r\u0000a\u0000p\u0000h\u0000 \u0000P\u0000r\u0000o\u0000p\u0000e\u0000r\u0000t\u0000y\u0000", "Æ[¦^þVhˆ^\\'`", "\u0000¼Ä³ø­|·\u0004ÕÁ1Á"]] string[][] [["C\u0000h\u0000a\u0000n\u0000n\u0000e\u0000l\u0000 \u0000E\u0000d\u0000i\u0000t\u0000o\u0000r\u0000", "\u001aS\u0016", "µÑ\\¸¸ÓÑÉ"]] string[][] [["C\u0000a\u0000l\u0000i\u0000b\u0000r\u0000a\u0000t\u0000i\u0000o\u0000n\u0000 \u0000P\u0000a\u0000r\u0000a\u0000m\u0000e\u0000t\u0000e\u0000r\u0000s\u0000 \u0000T\u0000a\u0000b\u0000l\u0000e\u0000", "!hÆQÂSpehˆ", "P­\u0000É\fÓ|·Tº0Ñ\\Ô"], ["M\u0000i\u0000c\u0000r\u0000o\u0000p\u0000h\u0000o\u0000n\u0000e\u0000 \u0000C\u0000a\u0000l\u0000i\u0000b\u0000r\u0000a\u0000t\u0000i\u0000o\u0000n\u0000", "¦žKQÎ˜!hÆQ", "È¹tÇlÐP­\u0000É"], ["U\u0000n\u0000i\u0000t\u0000s\u0000 \u0000S\u0000e\u0000t\u0000u\u0000p\u0000", "USMO¾‹š[", "è²\u0004Ç$Á\u0015È"], ["S\u0000i\u0000g\u0000n\u0000a\u0000l\u0000 \u0000T\u0000y\u0000p\u0000e\u0000 \u0000S\u0000e\u0000l\u0000e\u0000c\u0000t\u0000i\u0000o\u0000n\u0000", "áO÷S{|W\téb", "àÂ8Ö\u0015ÖÜÐ \u0000 ÁÝÐ"]] string[][] [["T\u0000e\u0000x\u0000t\u0000 \u0000p\u0000r\u0000e\u0000f\u0000e\u0000r\u0000e\u0000n\u0000c\u0000e\u0000", "e,g\u0018O\t", "ø¼8»°Æ Á ÁÝÐ"]] string[][] [["S\u0000t\u0000i\u0000m\u0000u\u0000l\u0000u\u0000s\u0000 \u0000E\u0000d\u0000i\u0000t\u0000o\u0000r\u0000", "Ào±R\u0016", "Çù­àÂ8Ö¸ÓÑÉ0®"]] string[][] [["H\u0000a\u0000r\u0000m\u0000o\u0000n\u0000i\u0000c\u0000 \u0000L\u0000i\u0000s\u0000t\u0000 \u0000E\u0000d\u0000i\u0000t\u0000o\u0000r\u0000", "\u0010âl\u0017Rh\u0016", "0¼pÈ\fÓ©º]¸ \u0000¸ÓÑÉ"]] string[][] [["S\u0000e\u0000a\u0000r\u0000c\u0000h\u0000 \u0000R\u0000a\u0000n\u0000g\u0000e\u0000 \u0000E\u0000d\u0000i\u0000t\u0000o\u0000r\u0000", "\u001cd\"}\u0003ôV\u0016", "ÐÐÉÀ”¼\u0004Ç¸ÓÑÉ"], ["U\u0000s\u0000e\u0000r\u0000 \u0000E\u0000q\u0000u\u0000a\u0000t\u0000i\u0000o\u0000n\u0000 \u0000P\u0000a\u0000r\u0000a\u0000m\u0000e\u0000t\u0000e\u0000r\u0000s\u0000 \u0000T\u0000a\u0000b\u0000l\u0000e\u0000", "(u7b¹e\u000bzÂSpehˆ", "¬À©ÆÇ)¼\u0015ÈÝÂÀ¼\u0018Â\\Ô"]] string[][] [["R\u0000e\u0000p\u0000l\u0000a\u0000c\u0000e\u0000 \u0000e\u0000x\u0000i\u0000s\u0000t\u0000i\u0000n\u0000g\u0000 \u0000F\u0000i\u0000l\u0000e\u0000?\u0000", "¤Nÿf†Nò]X[(W„v‡eöN\u0017T?\u0000", "tÇø» \u0000ˆÇ”² \u0000\fÓ|ÇDÇ \u0000P­´ÌXÕ ¬µÂÈ²L®?\u0000"], ["P\u0000l\u0000e\u0000a\u0000s\u0000e\u0000 \u0000e\u0000n\u0000t\u0000e\u0000r\u0000 \u0000a\u0000 \u0000n\u0000a\u0000m\u0000e\u0000", "÷eQ\rTW[", "tÇ„¹DÇ \u0000…Ç%¸XÕíÂÜÂ$Æ.\u0000"], ["E\u0000n\u0000t\u0000e\u0000r\u0000 \u0000c\u0000o\u0000m\u0000m\u0000e\u0000n\u0000t\u0000 \u0000f\u0000o\u0000r\u0000 \u0000d\u0000a\u0000t\u0000a\u0000f\u0000i\u0000l\u0000e\u0000:\u0000", "eQeöNèlã.\u0000", "ÇÌ¸\fÓ|ÇXÇ \u0000üÈtÕ|¹ \u0000Ç%¸XÕíÂÜÂ$Æ.\u0000"]] string[][] [["I\u0000n\u0000p\u0000u\u0000t\u0000 \u0000S\u0000e\u0000r\u0000i\u0000a\u0000l\u0000 \u0000N\u0000o\u0000", "eQ^\u0017R÷S", "Ä¬,¸ˆ¼8Ö…Ç%¸"]] string[][] [["N\u0000u\u0000m\u0000b\u0000e\u0000r\u0000 \u0000F\u0000o\u0000r\u0000m\u0000a\u0000t\u0000", "penc<h\u000f_", "\u0012¬$Á\u0015È"], ["A\u0000d\u0000d\u0000 \u0000C\u0000u\u0000r\u0000v\u0000e\u0000 \u0000N\u0000a\u0000m\u0000e\u0000", " R\nNòf¿~\rTW[", "á¬ ÁtÇ„¹¨Ì\u0000¬"], ["I\u0000m\u0000p\u0000o\u0000r\u0000t\u0000 \u0000W\u0000i\u0000z\u0000a\u0000r\u0000d\u0000 \u0000p\u00001\u0000", "ü[eQ\u0011Tü[ \u00001\u0000", "ø¼8»\fÓ|Ç\\¸€½0Ñ \u0000…Çl­-\u0000x¬LÇ \u00001\u0000"], ["I\u0000m\u0000p\u0000o\u0000r\u0000t\u0000 \u0000W\u0000i\u0000z\u0000a\u0000r\u0000d\u0000 \u0000p\u00002\u0000", "ü[eQ\u0011Tü[ \u00002\u0000", "ø¼8»\fÓ|Ç\\¸€½0Ñ \u0000…Çl­-\u0000x¬LÇ \u00002\u0000"], ["I\u0000m\u0000p\u0000o\u0000r\u0000t\u0000 \u0000W\u0000i\u0000z\u0000a\u0000r\u0000d\u0000 \u0000p\u00003\u0000", "ü[eQ\u0011Tü[ \u00003\u0000", "ø¼8»\fÓ|Ç\\¸€½0Ñ \u0000…Çl­-\u0000x¬LÇ \u00003\u0000"]] string[][] [["S\u0000i\u0000g\u0000n\u0000a\u0000l\u0000 \u0000G\u0000e\u0000n\u0000e\u0000r\u0000a\u0000t\u0000o\u0000r\u0000", "áO÷SÑS\u001fuhV", "àÂ8Ö\u001c¼ÝÀ0®"]] string[][] [["M\u0000u\u0000l\u0000t\u0000i\u0000m\u0000e\u0000t\u0000e\u0000r\u0000 \u0000", "\u0007N(uhˆ", "Ì¹¥²!Î\u0015ÈÄ¬0®"]] string[][] [["S\u0000c\u0000o\u0000p\u0000e\u0000-\u0000F\u0000F\u0000T\u0000", ":yâlhV", "$Æ0Å\\¸¤ÂTÏ\u0004Õ"], ["S\u0000c\u0000o\u0000p\u0000e\u0000-\u0000F\u0000F\u0000T\u0000", "1\u0006Rg", "¤Â™Ó¸Òt¹„½\u001dÁ"]] string[][] [[" \u0000O\u0000c\u0000t\u0000a\u0000v\u0000e\u0000 \u0000R\u0000e\u0000a\u0000l\u0000 \u0000T\u0000i\u0000m\u0000e\u0000 \u0000A\u0000n\u0000a\u0000l\u0000y\u0000z\u0000e\u0000r\u0000", "\rP\u000bz\u0006RghV", "%ÆÀÐ\f¾ \u0000äÂÜÂ\u0004¬tÕ\u001dÁ"]] string[][] [["S\u0000e\u0000l\u0000e\u0000c\u0000t\u0000 \u0000S\u0000t\u0000a\u0000r\u0000t\u0000u\u0000p\u0000 \u0000C\u0000o\u0000n\u0000f\u0000i\u0000g\u0000u\u0000r\u0000a\u0000t\u0000i\u0000o\u0000n\u0000", "\téb/T¨RMn.\u0000", "äÂÜÂ\u0004¬ü¬\u001cÈ,¸XÖ½¬"]] string[][] [[""]]] -> w12
    tunnel: w2 -> [_ _ _ w20 w28 _ w35 _ w37 _ w42 _ w49 _ _ w53 _ _ _ _ _ _ _ _ _ _ _ _ _ _ _ _ _ _ _ _ _ _ _ _ _ _]
    tunnel: "No" -> [_ _ _ _ _ _ _ _ _ _ _ _ _ _ _ _ _ _ _ _ _ _ _ _ _ _ _ _ _ _ _ _ _ _ _ _ _ _ _ _ _ _]
    tunnel: [_ _ _ w25 _ _ _ _ _ _ _ _ _ _ _ _ _ _ _ _ _ _ _ _ _ _ _ _ _ _ _ _ _ _ _ _ _ _ _ _ _ _] -> w3
    tunnel: [_ _ _ w24 w27 _ w34 _ w38 _ w41 _ w48 _ _ w52 _ _ _ _ _ _ _ _ _ _ _ _ _ _ _ _ _ _ _ _ _ _ _ _ _ _] -> w7
    tunnel: [_ _ _ w23 w29 _ w32 _ _ _ w43 _ w46 _ _ w54 _ _ _ _ _ _ _ _ _ _ _ _ _ _ _ _ _ _ _ _ _ _ _ _ _ _] -> w8
    tunnel: [_ _ _ w19 _ _ _ _ _ _ _ _ _ _ _ _ _ _ _ _ _ _ _ _ _ _ _ _ _ _ _ _ _ _ _ _ _ _ _ _ _ _] -> w4
    frame "Main" {
      # "10"
    }
    frame "Main Init" {
    }
    frame "About" {
    }
    frame "Main Toolbar" {
      w21 = string[][] [["A\u0000d\u0000d\u0000 \u0000S\u0000t\u0000e\u0000p\u0000", "y˜îvûm R", "mÕ©º”Í\u0000¬"], ["S\u0000t\u0000o\u0000p\u0000", "\\Pbk", "\u0015ÈÀÉ"], ["C\u0000o\u0000n\u0000t\u0000.\u0000", "ç~í~", "Ä¬Á"], ["S\u0000t\u0000o\u0000p\u0000", "\\Pbk", "\u0015ÈÀÉ"], ["R\u0000e\u0000d\u0000o\u0000", "l}", "à¬hÎ"], ["T\u0000i\u0000m\u0000e\u0000", "öeô•", "ÜÂ\u0004¬"], ["P\u0000r\u0000o\u0000j\u0000e\u0000c\u0000t\u0000", "y˜îv¡{\u0006t", "ü¬\u001cÈ,¸"], ["C\u0000u\u0000r\u0000v\u0000e\u0000s\u0000 \u0000L\u0000i\u0000b\u0000r\u0000a\u0000r\u0000y\u0000", "òf¿~“^", "á¬ Á\u001cÁà¬"], ["V\u0000a\u0000l\u0000u\u0000e\u0000 \u0000L\u0000i\u0000b\u0000r\u0000a\u0000r\u0000y\u0000", "pe<P“^", "è²\u001cÂ\u0012¬\u001cÁà¬"], ["R\u0000e\u0000s\u0000u\u0000l\u0000t\u0000 \u0000L\u0000i\u0000b\u0000r\u0000a\u0000r\u0000y\u0000", "Ó~œg“^", "°¬ü¬\u0012¬\u001cÁà¬"], ["W\u0000a\u0000v\u0000e\u0000 \u0000L\u0000i\u0000b\u0000r\u0000a\u0000r\u0000y\u0000", "öeßWâl“^", "ÜÂ\u0004¬\fÓ\u0015Ö\u001cÁà¬"], ["S\u0000t\u0000e\u0000p\u0000 \u0000S\u0000e\u0000t\u0000u\u0000p\u0000", "yîv\u0016", "mÕ©º¸ÓÑÉ"], ["D\u0000a\u0000t\u0000a\u0000 \u0000V\u0000i\u0000e\u0000w\u0000", "þVhˆ", "ÇÌ¸ô¼0®"], ["D\u0000o\u0000c\u0000u\u0000m\u0000e\u0000n\u0000t\u0000", "‡e,g", "8»\u001cÁ"], ["S\u0000i\u0000g\u0000n\u0000a\u0000l\u0000 \u0000G\u0000e\u0000n\u0000e\u0000r\u0000a\u0000t\u0000o\u0000r\u0000", "áO÷SÑS\u001fuhV", "àÂ8Ö\u001c¼ÝÀ0®"], ["M\u0000u\u0000l\u0000t\u0000i\u0000m\u0000e\u0000t\u0000e\u0000r\u0000", "\u0007N(uhˆ", "Ì¹¥²!Î\u0015ÈÄ¬0®"], ["T\u0000i\u0000m\u0000e\u0000 \u0000s\u0000e\u0000r\u0000i\u0000e\u0000s\u0000", "öeô^\u0017R", "$Æ0Å\\¸¤ÂTÏ\u0004Õ"], ["F\u0000F\u0000T\u0000", ":yâlhV", "¤Â™Ó¸Òt¹tÕ\u001dÁ0®"], ["O\u0000c\u0000t\u0000a\u0000v\u0000e\u0000 \u0000R\u0000e\u0000a\u0000l\u0000 \u0000T\u0000i\u0000m\u0000e\u0000 \u0000A\u0000n\u0000a\u0000l\u0000y\u0000z\u0000e\u0000r\u0000", "\rP\u000bz\u0006RghV", "%ÆÀÐ\f¾ \u0000äÂÜÂ\u0004¬tÕ\u001dÁ"], ["S\u0000t\u0000a\u0000r\u0000t\u0000", "\u0000_ËY", "ÜÂ‘Ç"], ["L\u0000o\u0000t\u0000:\u0000", "ÁT\rT:\u0000", "ˆÔ…º:\u0000"], ["S\u0000/\u0000N\u0000:\u0000", "^÷S:\u0000", "ˆ¼8Ö:\u0000"], ["T\u0000e\u0000s\u0000t\u0000e\u0000d\u0000:\u0000", "KmՋ:\u0000", "€¬¬À:\u0000"], ["M\u0000a\u0000n\u0000u\u0000a\u0000l\u0000", "(u7b\u0007cWS", "$Á…º\u001cÁ"], ["H\u0000o\u0000m\u0000e\u0000 \u0000p\u0000a\u0000g\u0000e\u0000", "Qu˜", "HÖ˜ÓÀÉ"], ["A\u0000b\u0000o\u0000u\u0000t\u0000 \u0000u\u0000s\u0000", "sQŽN¾|ðX", "\u0004Õ\\¸ø­Œ·ÐÅ \u0000\u0000³XÕìÅ"], ["H\u0000a\u0000r\u0000d\u0000w\u0000a\u0000r\u0000e\u0000", "lxöN", "¥ÇXÎ$Á\u0015È"], ["C\u0000a\u0000l\u0000i\u0000b\u0000r\u0000a\u0000t\u0000i\u0000o\u0000n\u0000", "!hÆQ", "P­\u0000É"]]  # Button Label On
      w22 = string[][] [["A\u0000d\u0000d\u0000 \u0000S\u0000t\u0000e\u0000p\u0000", "y˜îvûm R", "mÕ©º”Í\u0000¬"], ["S\u0000t\u0000a\u0000r\u0000t\u0000", "\u0000_ËY", "ÜÂ‘Ç"], ["C\u0000o\u0000n\u0000t\u0000.\u0000", "ç~í~", "Ä¬Á"], ["L\u0000o\u0000o\u0000p\u0000", "Þí~", "(¸Á"], ["R\u0000e\u0000d\u0000o\u0000", "l}", "à¬hÎ"], ["T\u0000i\u0000m\u0000e\u0000", "öeô•", "ÜÂ\u0004¬"], ["P\u0000r\u0000o\u0000j\u0000e\u0000c\u0000t\u0000", "y˜îv¡{\u0006t", "ü¬\u001cÈ,¸"], ["C\u0000u\u0000r\u0000v\u0000e\u0000s\u0000 \u0000L\u0000i\u0000b\u0000r\u0000a\u0000r\u0000y\u0000", "òf¿~“^", "á¬ Á\u001cÁà¬"], ["V\u0000a\u0000l\u0000u\u0000e\u0000 \u0000L\u0000i\u0000b\u0000r\u0000a\u0000r\u0000y\u0000", "pe<P“^", "è²\u001cÂ\u0012¬\u001cÁà¬"], ["R\u0000e\u0000s\u0000u\u0000l\u0000t\u0000 \u0000L\u0000i\u0000b\u0000r\u0000a\u0000r\u0000y\u0000", "Ó~œg“^", "°¬ü¬\u0012¬\u001cÁà¬"], ["W\u0000a\u0000v\u0000e\u0000 \u0000L\u0000i\u0000b\u0000r\u0000a\u0000r\u0000y\u0000", "öeßWâl“^", "ÜÂ\u0004¬\fÓ\u0015Ö\u001cÁà¬"], ["S\u0000t\u0000e\u0000p\u0000 \u0000S\u0000e\u0000t\u0000u\u0000p\u0000", "yîv\u0016", "mÕ©º¸ÓÑÉ"], ["D\u0000a\u0000t\u0000a\u0000 \u0000V\u0000i\u0000e\u0000w\u0000", "þVhˆ", "ø­|·\u0004Õ"], ["D\u0000o\u0000c\u0000u\u0000m\u0000e\u0000n\u0000t\u0000", "‡e,g", "8»\u001cÁ¸ÓÑÉ"], ["S\u0000i\u0000g\u0000n\u0000a\u0000l\u0000 \u0000G\u0000e\u0000n\u0000e\u0000r\u0000a\u0000t\u0000o\u0000r\u0000", "áO÷SÑS\u001fuhV", "àÂ8Ö\u001c¼ÝÀ0®"], ["M\u0000u\u0000l\u0000t\u0000i\u0000m\u0000e\u0000t\u0000e\u0000r\u0000", "\u0007N(uhˆ", "Ì¹¥²!Î\u0015ÈÄ¬0®"], ["T\u0000i\u0000m\u0000e\u0000 \u0000s\u0000e\u0000r\u0000i\u0000e\u0000s\u0000", "öeô^\u0017R", "$Æ0Å\\¸¤ÂTÏ\u0004Õ"], ["F\u0000F\u0000T\u0000", ":yâlhV", "¤Â™Ó¸Òt¹tÕ\u001dÁ0®"], ["O\u0000c\u0000t\u0000a\u0000v\u0000e\u0000 \u0000R\u0000e\u0000a\u0000l\u0000 \u0000T\u0000i\u0000m\u0000e\u0000 \u0000A\u0000n\u0000a\u0000l\u0000y\u0000z\u0000e\u0000r\u0000", "\rP\u000bz\u0006RghV", "%ÆÀÐ\f¾ \u0000äÂÜÂ\u0004¬tÕ\u001dÁ"], ["P\u0000a\u0000u\u0000s\u0000e\u0000", "\\Pbk", "\u0015ÈÀÉ"], ["L\u0000o\u0000t\u0000:\u0000", "ÁT\rT:\u0000", "ˆÔ…º:\u0000"], ["S\u0000/\u0000N\u0000:\u0000", "^÷S:\u0000", "ˆ¼8Ö:\u0000"], ["T\u0000e\u0000s\u0000t\u0000e\u0000d\u0000:\u0000", "KmՋ:\u0000", "€¬¬À:\u0000"], ["M\u0000a\u0000n\u0000u\u0000a\u0000l\u0000", "(u7b\u0007cWS", "$Á…º\u001cÁ"], ["H\u0000o\u0000m\u0000e\u0000 \u0000p\u0000a\u0000g\u0000e\u0000", "Qu˜", "HÖ˜ÓÀÉ"], ["A\u0000b\u0000o\u0000u\u0000t\u0000 \u0000u\u0000s\u0000", "sQŽN¾|ðX", "\u0004Õ\\¸ø­Œ·ÐÅ \u0000\u0000³XÕìÅ"], ["H\u0000a\u0000r\u0000d\u0000w\u0000a\u0000r\u0000e\u0000", "lxöN", "¥ÇXÎ$Á\u0015È"], ["C\u0000a\u0000l\u0000i\u0000b\u0000r\u0000a\u0000t\u0000i\u0000o\u0000n\u0000", "!hÆQ", "P­\u0000É"]]  # Button Label Off
      w23 = string[] ["AddStep", "Start", "Seq Continue", "Continue", "Redo", "Elapsed", "Project", "Curve Lib", "Value Lib", "TF Lib", "Wave Lib", "Step Setup", "Data View", "Document", "SignalGen", "MultiMeter", "Oscillo", "Spectral", "RTA", "Pause", "Lot:", "S/N:", "Tested:", "Manual", "Company Site", "About", "SetHardware", "SetCalibration"]  # Control Name
      w26 = string[][] [["A\u0000d\u0000d\u0000 \u0000S\u0000t\u0000e\u0000p\u0000", "y˜îvûm R", "ü¬\u001cÈmÕ©ºDÇ \u0000”Í\u0000¬iÕÈ²ä²"], ["S\u0000t\u0000a\u0000r\u0000t\u0000", "\u0000_ËY", "ü¬\u001cÈ,¸DÇ \u0000äÂ‰ÕiÕÈ²ä²"], ["R\u0000u\u0000n\u0000 \u0000c\u0000o\u0000n\u0000t\u0000i\u0000n\u0000u\u0000e\u0000", "ç~í~", "ü¬\u001cÈ,¸DÇ \u0000Ä¬Á \u0000äÂÕiÕÈ²ä²"], ["R\u0000u\u0000n\u0000 \u0000L\u0000o\u0000o\u0000p\u0000", "Þí~", "ü¬\u001cÈ,¸DÇ \u0000(¸Á\u0001È<Ç\\¸ \u0000äÂÕiÕÈ²ä²"], ["R\u0000e\u0000d\u0000o\u0000", "l}", "¬¬ÀÖ\u0018Â|¹ \u0000É\u0000¬ÜÂ¤ÐÀÉ \u0000JÅà¬ \u0000ä²ÜÂ \u0000äÂÕiÕÈ²ä²"], ["T\u0000i\u0000m\u0000e\u0000", "öeô•", "äÂ‰ÕÜÂ\u0004¬DÇ \u0000\\ÔÜÂiÕÈ²ä²"], ["P\u0000r\u0000o\u0000j\u0000e\u0000c\u0000t\u0000", "y˜îv¡{\u0006t", "ü¬\u001cÈ,¸=Ì8» \u0000ô¼0®"], ["C\u0000u\u0000r\u0000v\u0000e\u0000s\u0000 \u0000L\u0000i\u0000b\u0000r\u0000a\u0000r\u0000y\u0000", "òf¿~“^", "á¬ Á\u001cÁà¬=Ì8» \u0000ô¼0®"], ["V\u0000a\u0000l\u0000u\u0000e\u0000 \u0000L\u0000i\u0000b\u0000r\u0000a\u0000r\u0000y\u0000", "pe<P“^", "è²\u001cÂ\u0012¬\u001cÁà¬=Ì8» \u0000ô¼0®"], ["R\u0000e\u0000s\u0000u\u0000l\u0000t\u0000 \u0000L\u0000i\u0000b\u0000r\u0000a\u0000r\u0000y\u0000", "Ó~œg“^", "°¬ü¬\u0012¬\u001cÁà¬=Ì8» \u0000ô¼0®"], ["W\u0000a\u0000v\u0000e\u0000 \u0000L\u0000i\u0000b\u0000r\u0000a\u0000r\u0000y\u0000", "öeßWâl“^", "ÜÂ\u0004¬\fÓ\u0015Ö\u001cÁà¬=Ì8» \u0000ô¼0®"], ["S\u0000t\u0000e\u0000p\u0000 \u0000S\u0000e\u0000t\u0000u\u0000p\u0000", "yîv\u0016", "mÕ©º¸ÓÑÉ=Ì8» \u0000ô¼0®"], ["D\u0000a\u0000t\u0000a\u0000 \u0000V\u0000i\u0000e\u0000w\u0000", "þVhˆ", "ÇÌ¸ô¼0®=Ì8» \u0000ô¼0®"], ["D\u0000o\u0000c\u0000u\u0000m\u0000e\u0000n\u0000t\u0000", "‡e,g", "8»\u001cÁ¸ÓÑÉ=Ì8» \u0000ô¼0®"], ["S\u0000i\u0000g\u0000n\u0000a\u0000l\u0000 \u0000G\u0000e\u0000n\u0000e\u0000r\u0000a\u0000t\u0000o\u0000r\u0000", "áO÷SÑS\u001fuhV", "àÂ8Ö\u001c¼ÝÀ0®=Ì8» \u0000ô¼0®"], ["M\u0000u\u0000l\u0000t\u0000i\u0000m\u0000e\u0000t\u0000e\u0000r\u0000", "\u0007N(uhˆ", "Ì¹¥²!Î\u0015ÈÄ¬0®=Ì8» \u0000ô¼0®"], ["T\u0000i\u0000m\u0000e\u0000 \u0000s\u0000e\u0000r\u0000i\u0000e\u0000s\u0000", "öeô^\u0017R", "$Æ0Å\\¸¤ÂTÏ\u0004Õ=Ì8» \u0000ô¼0®"], ["F\u0000F\u0000T\u0000", ":yâlhV", "¤Â™Ó¸Òt¹tÕ\u001dÁ=Ì8» \u0000ô¼0®"], ["O\u0000c\u0000t\u0000a\u0000v\u0000e\u0000 \u0000R\u0000e\u0000a\u0000l\u0000 \u0000T\u0000i\u0000m\u0000e\u0000 \u0000A\u0000n\u0000a\u0000l\u0000y\u0000z\u0000e\u0000r\u0000", "\rP\u000bz\u0006RghV", "%ÆÀÐ\f¾tÕ\u001dÁ=Ì8» \u0000ô¼0®"], ["P\u0000a\u0000u\u0000s\u0000e\u0000", "\\Pbk", "\u0015ÈÀÉ"], ["P\u0000r\u0000o\u0000d\u0000u\u0000c\u0000t\u0000 \u0000N\u0000a\u0000m\u0000e\u0000", "ÁT\rT", "ÁÀˆÔ…º"], ["S\u0000e\u0000r\u0000i\u0000a\u0000l\u0000 \u0000N\u0000u\u0000m\u0000b\u0000e\u0000r\u0000", "^÷S", "Ä¬,¸ˆ¼8Ö"], ["T\u0000e\u0000s\u0000t\u0000e\u0000d\u0000 \u0000c\u0000o\u0000u\u0000n\u0000t\u0000", "KmՋpe", "€¬¬À\u0018Â"], ["U\u0000s\u0000e\u0000r\u0000 \u0000M\u0000a\u0000n\u0000u\u0000a\u0000l\u0000", "(u7b\u0007cWS", "$Á…º\u001cÁ"], ["h\u0000t\u0000t\u0000p\u0000:\u0000/\u0000/\u0000w\u0000w\u0000w\u0000.\u0000g\u0000v\u0000s\u0000l\u0000a\u0000b\u0000.\u0000c\u0000o\u0000m\u0000/\u0000I\u0000n\u0000f\u0000o\u0000/\u0000A\u0000b\u0000o\u0000u\u0000t\u0000.\u0000a\u0000s\u0000p\u0000", "h\u0000t\u0000t\u0000p\u0000:\u0000/\u0000/\u0000w\u0000w\u0000w\u0000.\u0000g\u0000v\u0000s\u0000l\u0000a\u0000b\u0000.\u0000c\u0000o\u0000m\u0000/\u0000I\u0000n\u0000f\u0000o\u0000/\u0000A\u0000b\u0000o\u0000u\u0000t\u0000.\u0000a\u0000s\u0000p\u0000", "HÖ˜ÓÀÉ"], ["A\u0000b\u0000o\u0000u\u0000t\u0000", "sQŽN¾|ðX", "\u0004Õ\\¸ø­Œ·ÐÅ \u0000\u0000³XÕìÅ"], ["H\u0000a\u0000r\u0000d\u0000w\u0000a\u0000r\u0000e\u0000", "lxöN", "¥ÇXÎ$Á\u0015ÈDÇ \u0000ÄÉ‰ÕiÕÈ²ä².\u0000"], ["C\u0000a\u0000l\u0000i\u0000b\u0000r\u0000a\u0000t\u0000i\u0000o\u0000n\u0000", "!hÆQ", "P­\u0000ÉDÇ \u0000ÄÉ‰ÕiÕÈ²ä².\u0000"]]  # Button Tooltip
      # "20"
      # "22"
      # "20"
      # "5"
      n3 = Index Array(array=w21, index (col)=w20) -> (element=w19:string[])  [unwired: 1 in]
      n4 = Index Array(array=w22, index (col)=w20) -> (element=w25:string[])  [unwired: 1 in]
      n5 = Index Array(array=w26, index (col)=w20) -> (element=w24:string[])  [unwired: 1 in]
    }
    frame "Common Toolbar" {
      w29 = string[] []  # Control Name
      w30 = string[][] [["C\u0000l\u0000o\u0000s\u0000e\u0000", "sQí•", "ë²0®"], ["H\u0000i\u0000d\u0000e\u0000 \u0000A\u0000u\u0000t\u0000o\u0000", "ê¨RÏ", "=Ì8»ÇÙ³(Â0®0®"], ["F\u0000i\u0000x\u0000", "úVš[", "=Ì8»à¬\u0015È"]]  # Button Tooltip
      n6 = Index Array(array=w30, index (col)=w28) -> (element=w27:string[])  [unwired: 1 in]
    }
    frame "Project" {
    }
    frame "Project Toolbar" {
      w32 = string[] ["TS Name", "Move Down", "Move Up", "Remove", "Property seq", "Property step", "ConfigureShowOnOff", "Expand/Collapse"]  # Control Name
      w33 = string[][] [["T\u0000a\u0000s\u0000k\u0000 \u0000S\u0000e\u0000q\u0000u\u0000e\u0000n\u0000c\u0000e\u0000s\u0000", "þ‹˜˜", "ü¬\u001cÈ,¸"], ["M\u0000o\u0000v\u0000e\u0000 \u0000D\u0000o\u0000w\u0000n\u0000", "ûy¨R\u0011T\u000bN", "mÕ©ºDÇ \u0000DÅ˜·\\¸ \u0000tÇÙ³"], ["M\u0000o\u0000v\u0000e\u0000 \u0000U\u0000p\u0000", "ûy¨R\u0011T\nN", "mÕ©ºDÇ \u0000°Æ\\¸ \u0000tÇÙ³"], ["D\u0000e\u0000l\u0000e\u0000t\u0000e\u0000 \u0000I\u0000t\u0000e\u0000m\u0000", "y˜îv Rd–", "mÕ©º \u0000­À\u001cÈ"], ["T\u0000a\u0000s\u0000k\u0000 \u0000S\u0000e\u0000q\u0000u\u0000e\u0000n\u0000c\u0000e\u0000 \u0000P\u0000r\u0000o\u0000p\u0000e\u0000r\u0000t\u0000y\u0000", "þ'`(", "ü¬\u001cÈ,¸ \u0000Á1Á"], ["S\u0000t\u0000e\u0000p\u0000 \u0000P\u0000r\u0000o\u0000p\u0000e\u0000r\u0000t\u0000y\u0000", "ek¤'`(", "mÕ©º \u0000Á1Á"], ["C\u0000o\u0000n\u0000f\u0000i\u0000g\u0000u\u0000r\u0000e\u0000S\u0000h\u0000o\u0000w\u0000O\u0000n\u0000O\u0000f\u0000f\u0000", "Ó~„g>f:y\u0000_/\u0000sQ", "l­1Áô¼0®/\u0000(Â0®0®"], ["E\u0000x\u0000p\u0000a\u0000n\u0000d\u0000/\u0000C\u0000o\u0000l\u0000l\u0000a\u0000p\u0000s\u0000e\u0000", "U\\\u0000_/\u00006eÞV", "¼ÓXÎ0®/\u0000\u0011È0®"]]  # Button Tooltip
      n7 = Index Array(array=w33, index (col)=w35) -> (element=w34:string[])  [unwired: 1 in]
    }
    frame "Curves Library" {
      # "13"
      # "12"
      # "11"
      # "10"
    }
    frame "Curves Library Toolbar" {
      n8 = Index Array(array=string[][] [["O\u0000p\u0000e\u0000n\u0000", "Sb\u0000_", "ôÅ0®"], ["S\u0000a\u0000v\u0000e\u0000", "ÝOX[", "ô¼\u0000­"], ["D\u0000e\u0000l\u0000e\u0000t\u0000e\u0000", " Rd–", "ÇÌ¸ÀÉ°Æ0®"], ["P\u0000r\u0000o\u0000t\u0000e\u0000c\u0000t\u0000", "ÝO¤b", "ÇÌ¸ô¼8Ö"], ["U\u0000n\u0000p\u0000r\u0000o\u0000t\u0000e\u0000c\u0000t\u0000", "ÖSˆmÝO¤b", "ÇÌ¸ô¼8ÖtÕ\u001cÈ"], ["A\u0000u\u0000t\u0000o\u0000P\u0000r\u0000o\u0000t\u0000e\u0000c\u0000t\u0000", "ê¨RÝO¤b", "ÇÙ³ÇÌ¸ô¼8Ö"], ["U\u0000n\u0000d\u0000o\u0000A\u0000u\u0000t\u0000o\u0000P\u0000r\u0000o\u0000t\u0000e\u0000c\u0000t\u0000", "ÖSmê¨RÝO¤b", "ÇÙ³ÇÌ¸ô¼8ÖtÕ\u001cÈ"], ["C\u0000o\u0000m\u0000p\u0000l\u0000e\u0000t\u0000e\u0000D\u0000e\u0000l\u0000e\u0000t\u0000e\u0000", " Rd–", "ÇÌ¸ÀÉ°Æ0®"]], index (col)=w37) -> (element=w38:string[])  [unwired: 1 in]
    }
    frame "Add Step" {
    }
    frame "Add Step Toolbar" {
      w43 = string[] ["Refresh", "Remove", "Option"]  # Control Name
      w44 = string[][] [["R\u0000e\u0000f\u0000r\u0000e\u0000s\u0000h\u0000", "7R°e", "ä²ÜÂ}Ç0®"], ["R\u0000e\u0000m\u0000o\u0000v\u0000e\u0000", " Rd–", "­À\u001cÈ"], ["O\u0000p\u0000t\u0000i\u0000o\u0000n\u0000", "\ty", "XÖ½¬$Á\u0015È"]]  # Button Tooltip
      n9 = Index Array(array=w44, index (col)=w42) -> (element=w41:string[])  [unwired: 1 in]
    }
    frame "Step Setup" {
    }
    frame "Step Setup Toolbar", "ViewData Toolbar" {
      w46 = string[] ["Load", "Save As", "Revert", "Property", "TitleShowOnOff", "LegendShowOnOff", "CursorShowOnOff", "PreviewShowOnOff", "Wave", "XY", "Polar", "Table", "Result", "Octave", "Text", "Digital", "Picture", "Intensity", "X_Autoscale", "Y1_Autoscale", "Y2_Autoscale", "Align"]  # Control Name
      w47 = string[][] [["O\u0000p\u0000e\u0000n\u0000", "Sb\u0000_", "mÕ©ºôÅ0®"], ["S\u0000a\u0000v\u0000e\u0000 \u0000A\u0000s\u0000", "æSX[:N", "mÕ©ºDÇ \u0000tÇ„¹DÇ \u0000\u0014¼¸¯´Å \u0000ô¼\u0000­"], ["R\u0000e\u0000v\u0000e\u0000r\u0000t\u0000", "b`\rY", "ÇÌ¸Öõ¼"], ["P\u0000r\u0000o\u0000p\u0000e\u0000r\u0000t\u0000y\u0000", "'`(", "ø­|·\u0004ÕÁ1Á"], ["T\u0000i\u0000t\u0000l\u0000e\u0000 \u0000S\u0000h\u0000o\u0000w\u0000 \u0000O\u0000n\u0000/\u0000O\u0000f\u0000f\u0000", "\u0007h˜˜>f:y\u0000_/\u0000sQ", "\\Ô\u001cÈ`·ô¼0®/\u0000(Â0®0®"], ["L\u0000e\u0000g\u0000e\u0000n\u0000d\u0000S\u0000h\u0000o\u0000w\u0000O\u0000n\u0000O\u0000f\u0000f\u0000", "þV‹O>f:y\u0000_/\u0000sQ", "tÇ„¹©º]¸ \u0000\\ÔÜÂ/\u0000(Â0®0®"], ["C\u0000u\u0000r\u0000s\u0000o\u0000r\u0000S\u0000h\u0000o\u0000w\u0000O\u0000n\u0000O\u0000f\u0000f\u0000", "8n\u0007h>f:y\u0000_/\u0000sQ", " Ç\\Ô=Ì8» \u0000\\ÔÜÂ/\u0000(Â0®0®"], ["P\u0000r\u0000e\u0000v\u0000i\u0000e\u0000w\u0000S\u0000h\u0000o\u0000w\u0000O\u0000n\u0000O\u0000f\u0000f\u0000", "„˜È‰>f:y\u0000_/\u0000sQ", "ø»¬¹ô¼0®=Ì8» \u0000\\ÔÜÂ/\u0000(Â0®0®"], ["A\u0000d\u0000d\u0000 \u0000W\u0000a\u0000v\u0000e\u0000 \u0000G\u0000r\u0000a\u0000p\u0000h\u0000", "âlþVhˆÒceQ", "ÜÂ\u0004¬\fÓ\u0015Öø­|·\u0004Õ \u0000”Í\u0000¬"], ["A\u0000d\u0000d\u0000 \u0000X\u0000Y\u0000 \u0000G\u0000r\u0000a\u0000p\u0000h\u0000", "X\u0000Y\u0000þVhˆÒceQ", "X\u0000Y\u0000ø­|·\u0004Õ \u0000”Í\u0000¬"], ["A\u0000d\u0000d\u0000 \u0000P\u0000o\u0000l\u0000a\u0000r\u0000 \u0000G\u0000r\u0000a\u0000p\u0000h\u0000", "gPW\u0007hþVhÒceQ", "ù­Ç¬¹\\Ôø­|·\u0004Õ \u0000Í\u0000¬"], ["A\u0000d\u0000d\u0000 \u0000T\u0000a\u0000b\u0000l\u0000e\u0000", "hˆÒceQ", "\\Ô \u0000”Í\u0000¬"], ["A\u0000d\u0000d\u0000 \u0000R\u0000e\u0000s\u0000u\u0000l\u0000t\u0000", "Ó~œgÒceQ", "°¬ü¬\u0012¬ \u0000”Í\u0000¬"], ["A\u0000d\u0000d\u0000 \u0000O\u0000c\u0000t\u0000a\u0000v\u0000e\u0000 \u0000G\u0000r\u0000a\u0000p\u0000h\u0000", "\rP‘˜\u000bzþVhˆÒceQ", "%ÆÀÐ\f¾ø­|·\u0004Õ \u0000”Í\u0000¬"], ["A\u0000d\u0000d\u0000 \u0000T\u0000e\u0000x\u0000t\u0000", ",g‡eÒceQ", "ø¼8» \u0000”Í\u0000¬"], ["A\u0000d\u0000d\u0000 \u0000D\u0000i\u0000g\u0000i\u0000t\u0000a\u0000l\u0000 \u0000G\u0000r\u0000a\u0000p\u0000h\u0000", "peW[þVhˆÒceQ", "\u0018ÂÇàÂ8Öø­|·\u0004Õ \u0000Í\u0000¬"], ["A\u0000d\u0000d\u0000 \u0000P\u0000i\u0000c\u0000t\u0000u\u0000r\u0000e\u0000", "þVÏPÒceQ", "ø­¼¹ \u0000”Í\u0000¬"], ["A\u0000d\u0000d\u0000 \u0000I\u0000n\u0000t\u0000e\u0000n\u0000s\u0000i\u0000t\u0000y\u0000 \u0000G\u0000r\u0000a\u0000p\u0000h\u0000", "Æ[¦^þVhˆÒceQ", "\u0000¼Ä³ø­|·\u0004Õ \u0000”Í\u0000¬"], ["X\u0000_\u0000A\u0000u\u0000t\u0000o\u0000s\u0000c\u0000a\u0000l\u0000e\u0000", "X\u0000t \u0000ê¨R/\u0000Kb¨R", "X\u0000Í \u0000ÇÙ³/\u0000\u0018ÂÙ³"], ["Y\u00001\u0000_\u0000A\u0000u\u0000t\u0000o\u0000s\u0000c\u0000a\u0000l\u0000e\u0000", "Y\u00001\u0000t \u0000ê¨R/\u0000Kb¨R", "Y\u00001\u0000Í \u0000ÇÙ³/\u0000\u0018ÂÙ³"], ["Y\u00002\u0000_\u0000A\u0000u\u0000t\u0000o\u0000s\u0000c\u0000a\u0000l\u0000e\u0000", "Y\u00002\u0000t \u0000ê¨R/\u0000Kb¨R", "Y\u00002\u0000Í \u0000ÇÙ³/\u0000\u0018ÂÙ³"], ["G\u0000r\u0000a\u0000p\u0000h\u0000 \u0000W\u0000i\u0000n\u0000d\u0000o\u0000w\u0000 \u0000A\u0000l\u0000i\u0000g\u0000n\u0000", "—zãSù[PŸ", "=Ì8»\u0015È,¸"]]  # Button Tooltip
      n10 = Index Array(array=w47, index (col)=w49) -> (element=w48:string[])  [unwired: 1 in]
    }
    frame "ViewData" {
    }
    frame "Document" {
    }
    frame "Document Toolbar" {
      w54 = string[] ["BtnOpen", "Combo Box", "BtnSave", "BtnPrint", "BtnPage", "BtnImage", "BtnLot", "BtnSN", "BtnDATE"]  # Control Name
      w55 = string[][] [["O\u0000p\u0000e\u0000n\u0000", "Sb\u0000_", "8»\u001cÁôÅ0®"], ["E\u0000x\u0000p\u0000o\u0000r\u0000t\u0000 \u0000F\u0000i\u0000l\u0000e\u0000 \u0000F\u0000o\u0000r\u0000m\u0000a\u0000t\u0000", "úQeöN<h\u000f_", "\fÓ|Çô¼\u0000­\u0015ÖÝÂ"], ["E\u0000x\u0000p\u0000o\u0000r\u0000t\u0000", "úQ", "8»\u001cÁœÍl­"], ["P\u0000r\u0000i\u0000n\u0000t\u0000", "SbpS", "xÇÄÁ"], ["P\u0000a\u0000g\u0000e\u0000 \u0000S\u0000e\u0000t\u0000u\u0000p\u0000", "u˜b—¾‹n", "˜ÓÀÉ$Á\u0015È"], ["I\u0000n\u0000s\u0000e\u0000r\u0000t\u0000 \u0000P\u0000i\u0000c\u0000t\u0000u\u0000r\u0000e\u0000", "ÒceQþVÏP", "ø­¼¹½À…Ç"], ["I\u0000n\u0000s\u0000e\u0000r\u0000t\u0000 \u0000P\u0000r\u0000o\u0000d\u0000u\u0000c\u0000t\u0000 \u0000N\u0000a\u0000m\u0000e\u0000", "ÒceQÁTLr", "ÁÀˆÔ…º½À…Ç"], ["I\u0000n\u0000s\u0000e\u0000r\u0000t\u0000 \u0000S\u0000N\u0000", "ÒceQ^÷S", "Ä¬,¸ˆ¼8Ö½À…Ç"], ["I\u0000n\u0000s\u0000e\u0000r\u0000t\u0000 \u0000D\u0000a\u0000t\u0000e\u0000/\u0000T\u0000i\u0000m\u0000e\u0000", "ÒceQåe\u001fgöeô•", " °ÇÜÂ\u0004¬½ÀÇ"]]  # Button Tooltip
      n11 = Index Array(array=w55, index (col)=w53) -> (element=w52:string[])  [unwired: 1 in]
    }
    frame "Run Project" {
    }
    frame "WAVE" {
    }
    frame "XY" {
    }
    frame "DIGITAL" {
    }
    frame "OCTAVE" {
    }
    frame "POLAR" {
    }
    frame "TEXT" {
    }
    frame "TABLE" {
    }
    frame "PICTURE" {
    }
    frame "RESULT" {
    }
    frame "INTENSITY" {
    }
    frame "Hardware" {
    }
    frame "Calibration" {
    }
    frame "Messages" {
    }
    frame "Stimulus" {
    }
    frame "Analysis" {
    }
    frame "Post Processing" {
    }
    frame "Auto Save" {
    }
    frame "Serial No" {
    }
    frame "Recall" {
    }
    frame "Signal Generator" {
    }
    frame "Multimeter" {
    }
    frame "Oscilloscope-FFT" {
    }
    frame "RTA" {
    }
    frame "Operator Configure" {
    }
    frame Default {
    }
  }
  "Control Label On" <- w3
  "Control Name" <- w8
  "Control Label Off" <- w4
  n12 = Index Array(array=w12, index (row)="No", index (col)=w2) -> (element=w9:string)
  "Unicode String" <- w9
  n13 = case shown="\"Chinese traditional\"" w1 {
    tunnel: [w82 w83 w84 w85] -> w6
    frame "English", Default {
      w82 = u32 0 items=["System default"=0, "Latin-1"=1252, "Japanese"=932, "Korean"=947, "Chinese simplified"=936, "Chinese traditional"=950, "Central Europe"=1250, "Cyrillic"=1251, "Greek"=1253, "Turkish"=1254, "Hebrew"=1255, "Arabic"=1256, "Baltic"=1257, "Thai"=874, "Vietnamese"=783, "UTF8"=65001, "UTF-7"=65000] ("Code Page")
    }
    frame "Chinese traditional" {
      w83 = u32 950 items=["System default"=0, "Latin-1"=1252, "Japanese"=932, "Korean"=947, "Chinese simplified"=936, "Chinese traditional"=950, "Central Europe"=1250, "Cyrillic"=1251, "Greek"=1253, "Turkish"=1254, "Hebrew"=1255, "Arabic"=1256, "Baltic"=1257, "Thai"=874, "Vietnamese"=783, "UTF8"=65001, "UTF-7"=65000] ("Code Page")
    }
    frame "Chinese" {
      w84 = u32 936 items=["System default"=0, "Latin-1"=1252, "Japanese"=932, "Korean"=947, "Chinese simplified"=936, "Chinese traditional"=950, "Central Europe"=1250, "Cyrillic"=1251, "Greek"=1253, "Turkish"=1254, "Hebrew"=1255, "Arabic"=1256, "Baltic"=1257, "Thai"=874, "Vietnamese"=783, "UTF8"=65001, "UTF-7"=65000] ("Code Page")
    }
    frame "Korean" {
      w85 = u32 949 items=["System default"=0, "Latin-1"=1252, "Japanese"=932, "Korean"=949, "Chinese simplified"=936, "Chinese traditional"=950, "Central Europe"=1250, "Cyrillic"=1251, "Greek"=1253, "Turkish"=1254, "Hebrew"=1255, "Arabic"=1256, "Baltic"=1257, "Thai"=874, "Vietnamese"=783, "UTF8"=65001, "UTF-7"=65000] ("Code Page")
    }
  }
  n14 = for {
    tunnel: w7 -> [w87] mode=indexing
    tunnel: w6 -> [w88]
    tunnel: [w86] -> w5 mode=indexing
    n15 = call "GVSConvert Unicode to Multibyte.vi"("Code Page"=w88, "Unicode String"=w87) -> ("Multibyte string"=w86:string)  [unwired: 8 in, 1 out]
  }
  "Tip Strip" <- w5
  n16 = call "GVSConvert Unicode to Multibyte.vi"("Code Page"=w6, "Unicode String"=w9) -> ("Multibyte string"=→"Multibyte String":string)  [unwired: 8 in, 1 out]
